vi "总磷总氮通讯.vi"() -> ()   [LabVIEW 2016, in "斯坦道总磷总氮.lvlib"]
uses:
  <vilib>/Plasmionique/MB Master/MB_Master_Serial/MB_Master_Serial.lvclass
  C:/Program Files (x86)/National Instruments/LabVIEW 2016/vi.lib/Plasmionique/MB Master/MB_Master/MB_Master.lvclass
  <vilib>/Plasmionique/MB Master/MB_Master_TCP/MB_Master_TCP.lvclass
  <vilib>/Utility/config.llb/Write Key (Boolean).vi
  <vilib>/Utility/config.llb/Write Key (String).vi
  <vilib>/Plasmionique/MB Master/MB_Master/MB_Master.lvclass
  <vilib>/Utility/config.llb/NI_LVConfig.lvlib
  <vilib>/Plasmionique/MB Master/MB Master.lvlib
  <vilib>/ptbypt/NI_PtbyPt.lvlib
panel:
  out "启用":bool=TRUE
  out "氨氮状态告警区":u16[](array[numeric])
  out "氨氮测量数据区":u16[](array[numeric])
  out "COD测量数据区":u16[](array[numeric])
  out "COD状态告警区":u16[](array[numeric])
  out "总氮测量数据区":u16[](array[numeric])
  out "总氮状态告警区":u16[](array[numeric])
  out "总磷状态告警区":u16[](array[numeric])
  out "总磷测量数据区":u16[](array[numeric])
  out "状态告警区":T1 {"告警代码" items=["无告警", "缺试剂告警", "缺水样告警", "缺蒸馏水告警", "缺标液告警", "仪表漏液告警", "标定异常告警", "超量程告警", "加热异常", "低试剂预警", "超上限告警", "超下限告警", "仪表内部其他异常", "滴定异常告警", "电极异常告警", "量程切换告警", "参数设置告警", "PH电极电位异常", "电导率电极异常", "浊度光度异常", "溶解氧电极异常", "溶解氧光强异常", "温度异常告警", "PH异常告警", "溶解氧异常告警", "电导率异常告警", "浊度异常告警", "叶绿素异常告警", "藻密度异常告警", "蓝绿藻异常告警", "ORP异常告警", "氨氮异常告警", "清洁刷异常告警", "SD卡异常告警", "蓝牙异常告警", "Wifi异常告警", "流程异常告警"]; "故障代码" items=["无故障", "电机故障", "温度故障", "通讯故障", "滴定故障"]}
  out "测量数据区":T2 {"单位" items=["ug/L", "mg/L", "ppm", "mg/m3", "cm", "ppb", "ug/m3", "%", "nmol/mol", "umol/mol", "MPN/L", "MPN/100ml", "ng/m3", "NTU", "无量纲", "ms/cm", "us/cm", "℃", "mV", "万个/L"]}
  out "status":bool
  out "关键参数区":T3
  in  "读关键参数区":bool
  in  "读状态告警区":bool
  in  "读测量数据区":bool
  in  "站号":u16(ring) items=["总磷"=1, "氨氮"=3]
  in  "停止":bool
  in  "启动":bool
  in  "控制命令":u16(ring) items=["启动测量"=1, "标样核查"=2, "零点核查"=3, "跨度核查"=4, "空白测试"=5, "平行样测试"=6, "加标回收"=7, "空白校准"=8, "标样校准"=9, "初始化（清洗）"=10, "停止测试"=11, "仪器重启"=12, "校时"=13, "模式设置"=14, "测量间隔设置"=15]
  in  "控制命令参数":u16[](array[numeric]) format="%04xH"
  in  "VISA Resource":refnum<visa-resource-name>
  in  "启用模块":bool
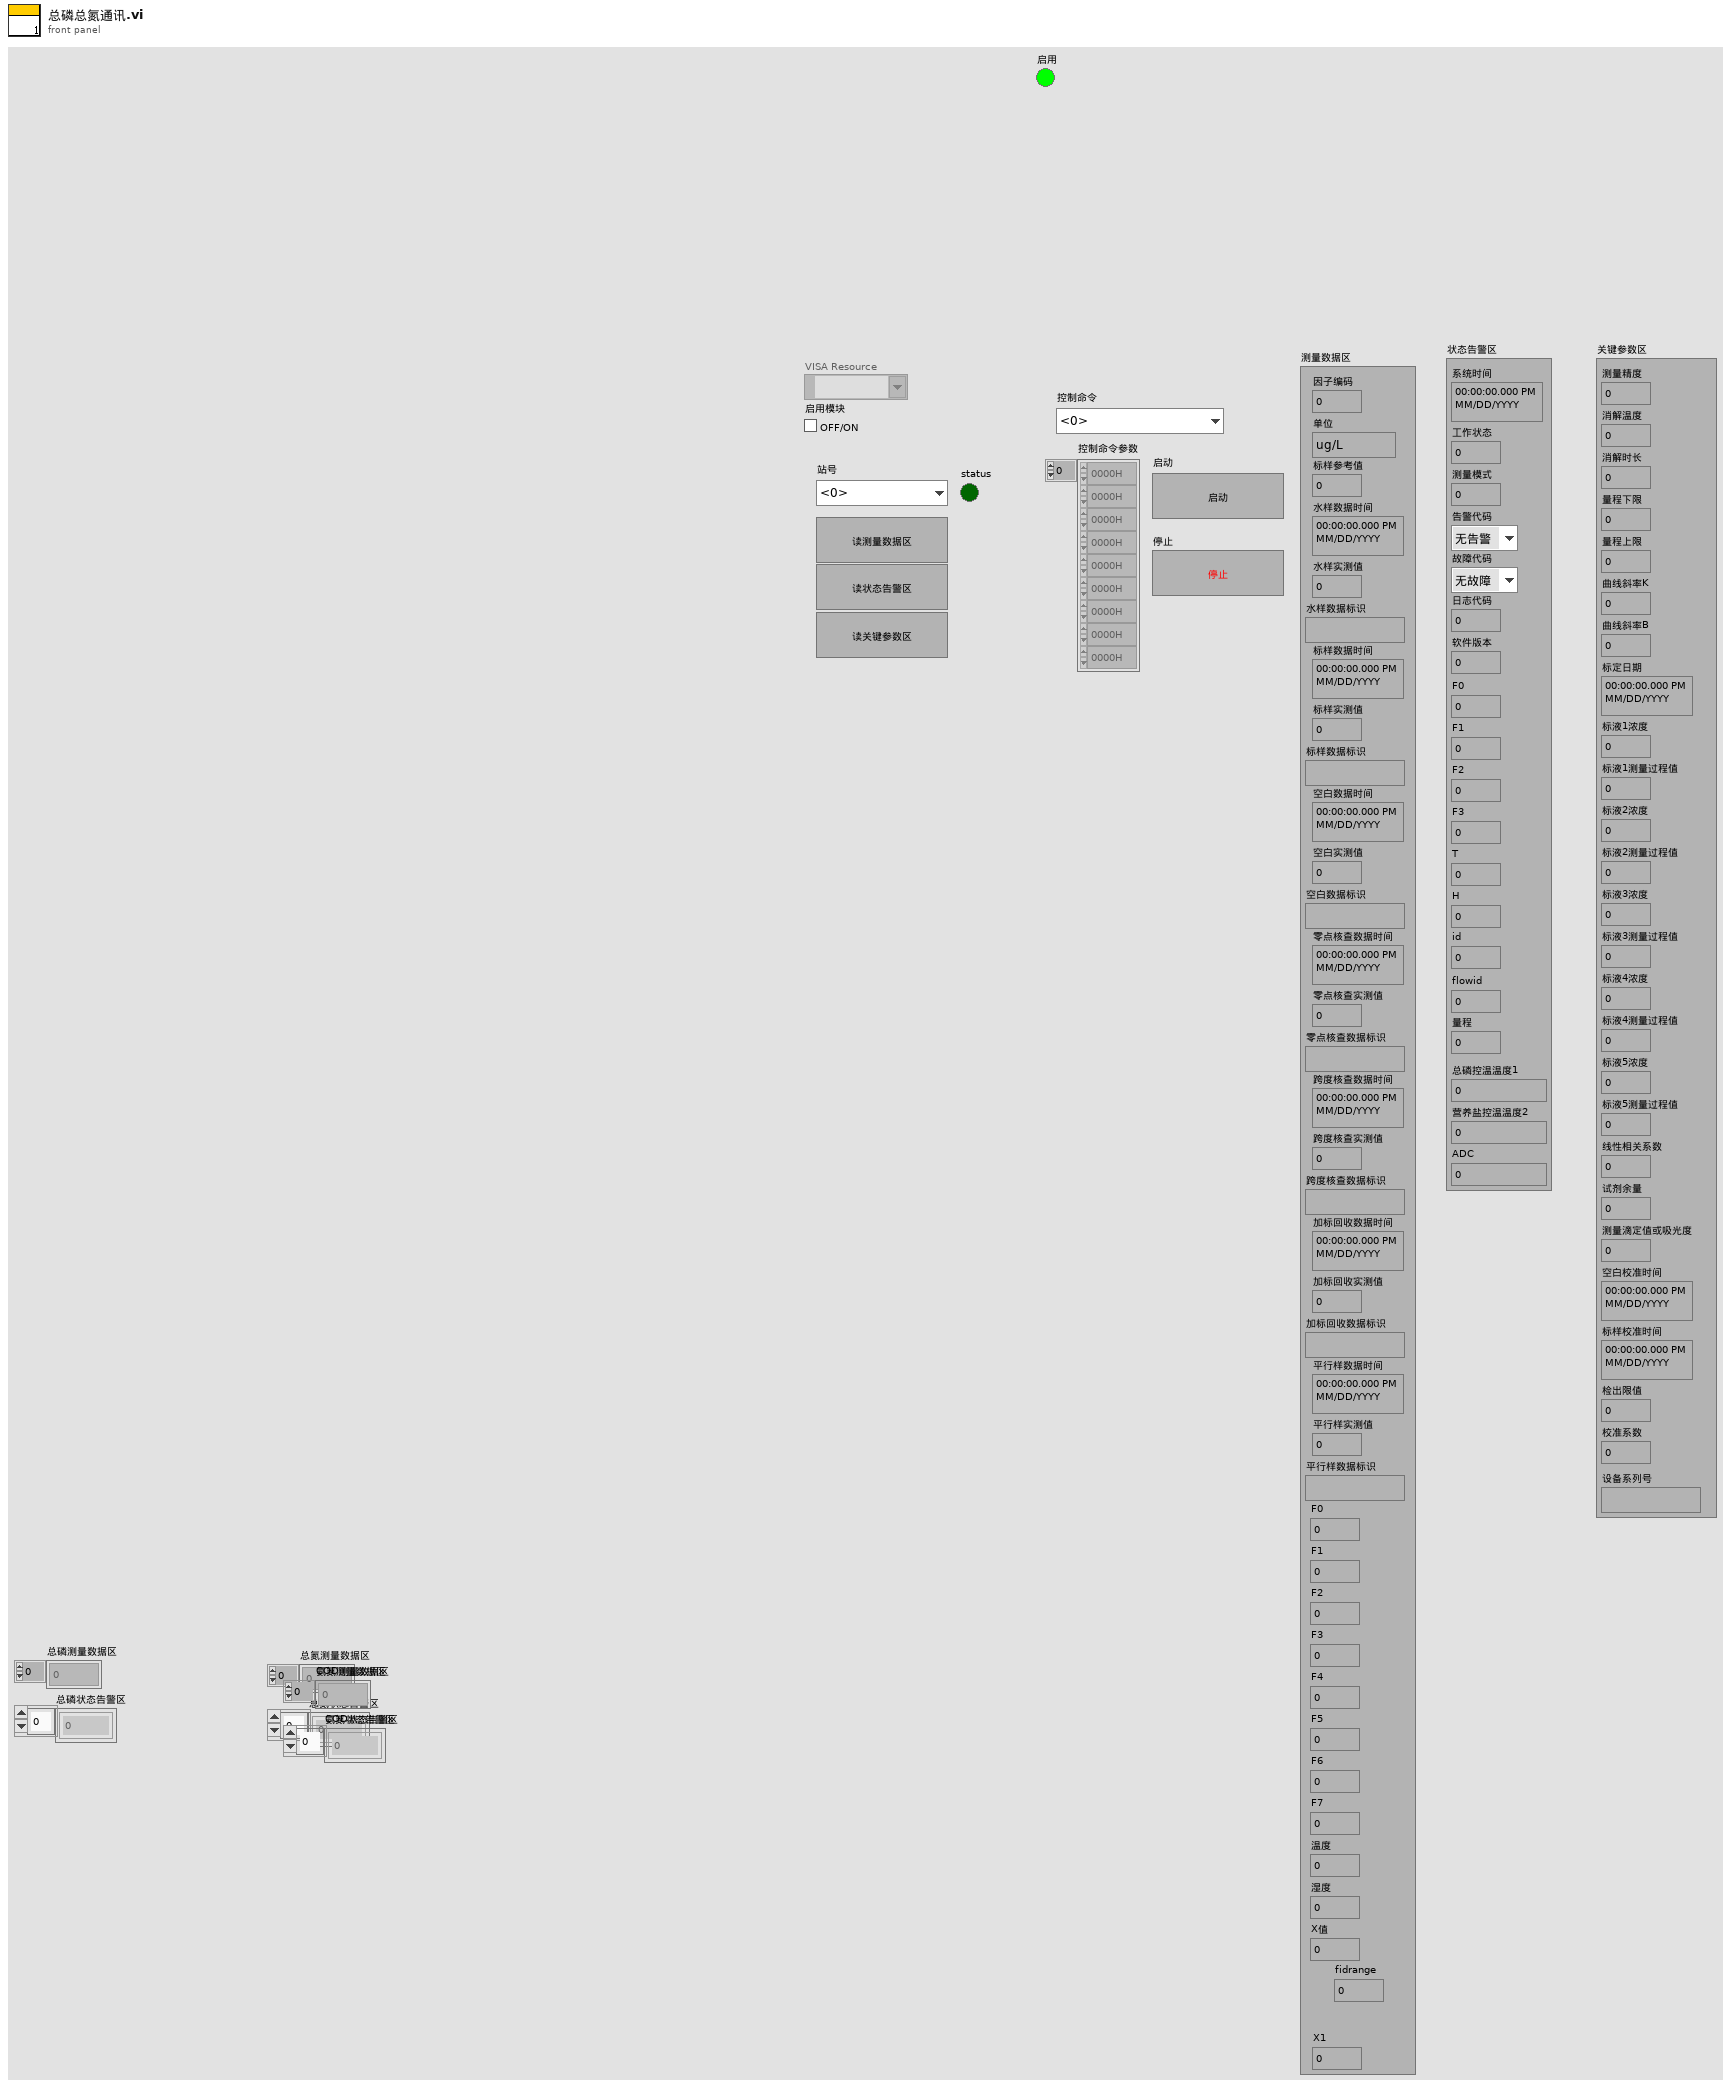
[diagram p1: front panel]
types:
  T1 = cluster{"系统时间":timestamp, "工作状态":u16, "测量模式":u16, "告警代码":u16, "故障代码":u16, "日志代码":u16, "软件版本":u16, "F0":sgl, "F1":sgl, "F2":sgl, "F3":sgl, "T":sgl, "H":sgl, "id":u16, "flowid":u16, "量程":u16, "总磷控温温度1":sgl, "营养盐控温温度2":sgl, "ADC":sgl}
  T2 = cluster{"因子编码":u32, "单位":u16, "标样参考值":sgl, "水样数据时间":timestamp, "水样实测值":sgl, "水样数据标识":string, "标样数据时间":timestamp, "标样实测值":sgl, "标样数据标识":string, "空白数据时间":timestamp, "空白实测值":sgl, "空白数据标识":string, "零点核查数据时间":timestamp, "零点核查实测值":sgl, "零点核查数据标识":string, "跨度核查数据时间":timestamp, "跨度核查实测值":sgl, "跨度核查数据标识":string, "加标回收数据时间":timestamp, "加标回收实测值":sgl, "加标回收数据标识":string, "平行样数据时间":timestamp, "平行样实测值":sgl, "平行样数据标识":string, "F0":sgl, "F1":sgl, "F2":sgl, "F3":sgl, "F4":sgl, "F5":sgl, "F6":sgl, "F7":sgl, "温度":sgl, "湿度":sgl, "X值":sgl, "fidrange":u16, "X1":sgl}
  T3 = cluster{"测量精度":u16, "消解温度":u16, "消解时长":u16, "量程下限":sgl, "量程上限":sgl, "曲线斜率K":sgl, "曲线斜率B":sgl, "标定日期":timestamp, "标液1浓度":sgl, "标液1测量过程值":sgl, "标液2浓度":sgl, "标液2测量过程值":sgl, "标液3浓度":sgl, "标液3测量过程值":sgl, "标液4浓度":sgl, "标液4测量过程值":sgl, "标液5浓度":sgl, "标液5测量过程值":sgl, "线性相关系数":sgl, "试剂余量":u32, "测量滴定值或吸光度":sgl, "空白校准时间":timestamp, "标样校准时间":timestamp, "检出限值":sgl, "校准系数":sgl, "设备系列号":string}
  T4 = cluster{"系统时间":timestamp, "工作状态":u16, "测量模式":enum16{"待机", "连续模式", "周期模式", "定点模式", "受控模式", "手动模式"}, "告警代码":u16, "故障代码":u16, "日志代码":u16, "软件版本":u16, "F0":sgl, "F1":sgl, "F2":sgl, "F3":sgl, "T":sgl, "H":sgl, "id":u16, "flowid":u16, "量程":u16, "总磷控温温度1":sgl, "营养盐控温温度2":sgl, "ADC":sgl}
  T5 = cluster{"因子编码":u32, "单位":u16, "标样参考值":sgl, "水样数据时间":timestamp, "水样实测值":sgl, "水样数据标识":string, "标样数据时间":timestamp, "标样实测值":sgl, "标样数据标识":string, "空白数据时间":timestamp, "空白实测值":sgl, "空白数据标识":string, "零点核查数据时间":timestamp, "零点核查实测值":sgl, "零点核查数据标识":string, "跨度核查数据时间":timestamp, "跨度核查实测值":sgl, "跨度核查数据标识":string, "加标回收数据时间":timestamp, "加标回收实测值":sgl, "加标回收数据标识":string, "平行样数据时间":timestamp, "平行样实测值":sgl, "平行样数据标识":string, "F0":sgl, "F1":sgl, "F2":sgl, "F3":sgl, "F4":sgl, "F5":sgl, "F6":sgl, "F7":sgl, "温度":sgl, "湿度":sgl, "X值":sgl, "fidrange":u16, "X1值":sgl}
  T6 = cluster{"测量精度":u16, "消解温度":u16, "消解时长":u16, "量程下限":sgl, "量程上限":sgl, "曲线斜率K":sgl, "曲线斜率B":sgl, "标定日期":timestamp, "标液1浓度":sgl, "标液1测量过程值":sgl, "标液2浓度":sgl, "标液2测量过程值":sgl, "标液3浓度":sgl, "标液3测量过程值":sgl, "标液4浓度":sgl, "标液4测量过程值":sgl, "标液5浓度":sgl, "标液5测量过程值":sgl, "线性相关系数":sgl, "试剂余量":u32, "测量滴定值或吸光度":sgl, "空白校准时间":timestamp, "标样校准时间":timestamp, "检出限值":sgl, "校准系数":sgl, "设备系列号":string}[]
  T7 = cluster{"系统时间":timestamp, "工作状态":u16, "测量模式":enum16{"待机", "连续模式", "周期模式", "定点模式", "受控模式", "手动模式"}, "告警代码":u16, "故障代码":u16, "日志代码":u16, "软件版本":u16, "F0":sgl, "F1":sgl, "F2":sgl, "F3":sgl, "T":sgl, "H":sgl, "id":u16, "flowid":u16, "量程":u16, "总磷控温温度1":sgl, "营养盐控温温度2":sgl, "ADC":sgl}[]
  T8 = cluster{"因子编码":u32, "单位":u16, "标样参考值":sgl, "水样数据时间":timestamp, "水样实测值":sgl, "水样数据标识":string, "标样数据时间":timestamp, "标样实测值":sgl, "标样数据标识":string, "空白数据时间":timestamp, "空白实测值":sgl, "空白数据标识":string, "零点核查数据时间":timestamp, "零点核查实测值":sgl, "零点核查数据标识":string, "跨度核查数据时间":timestamp, "跨度核查实测值":sgl, "跨度核查数据标识":string, "加标回收数据时间":timestamp, "加标回收实测值":sgl, "加标回收数据标识":string, "平行样数据时间":timestamp, "平行样实测值":sgl, "平行样数据标识":string, "F0":sgl, "F1":sgl, "F2":sgl, "F3":sgl, "F4":sgl, "F5":sgl, "F6":sgl, "F7":sgl, "温度":sgl, "湿度":sgl, "X值":sgl, "fidrange":u16, "X1值":sgl}[]
  T9 = typedef "CODCr交互.ctl" = cluster{"状态告警区":cluster{"系统时间":timestamp, "工作状态":u16, "测量模式":enum16{"待机", "连续模式", "周期模式", "定点模式", "受控模式", "手动模式"}, "告警代码":u16, "故障代码":u16, "日志代码":u16, "软件版本":u16, "F0":sgl, "F1":sgl, "F2":sgl, "F3":sgl, "T":sgl, "H":sgl, "id":u16, "flowid":u16, "量程":u16, "总磷控温温度1":sgl, "营养盐控温温度2":sgl, "ADC":sgl}, "平台试剂余量百分比":sgl, "关键参数":cluster{"测量量程":dbl, "测量精度":dbl, "测量间隔":dbl, "消解温度":dbl, "消解时长":dbl, "空白校准时间":timestamp, "曲线截距":dbl, "曲线斜率":dbl, "测量检出限":dbl, "测量信号值":dbl, "线性相关系数":dbl, "二次多项式系数":dbl, "标样校准时间":timestamp, "稀释倍数":dbl, "三项式系数":dbl, "空白标定系数":dbl, "量程系数":dbl, "F0/ORPA":dbl, "F1/ORPB":dbl, "F2/ORPK":dbl, "F3":dbl, "F4":dbl, "F5":dbl, "F6":dbl, "F7":dbl, "X0/滴定数":dbl, "量程":dbl}, "关键参数改变":bool, "校准信息":cluster{"低标液1浓度":dbl, "低标液1信号值":dbl, "低标液1启用":u16, "低标液2浓度":dbl, "低标液2信号值":dbl, "低标液2启用":u16, "低标液3浓度":dbl, "低标液3信号值":dbl, "低标液3启用":u16, "低标液4浓度":dbl, "低标液4信号值":dbl, "低标液4启用":u16, "低标液5浓度":dbl, "低标液5信号值":dbl, "低标液5启用":u16, "高标液1浓度":dbl, "高标液1信号值":dbl, "高标液1启用":u16, "高标液2浓度":dbl, "高标液2信号值":dbl, "高标液2启用":u16, "高标液3浓度":dbl, "高标液3信号值":dbl, "高标液3启用":u16, "高标液4浓度":dbl, "高标液4信号值":dbl, "高标液4启用":u16, "高标液5浓度":dbl, "高标液5信号值":dbl, "高标液5启用":u16, "低斜率":dbl, "低截距":dbl, "低二次多项式系数":dbl, "低线性相关系数":dbl, "高斜率":dbl, "高截距":dbl, "高二次多项式系数":dbl, "高线性相关系数":dbl}, "校准信息改变":bool}
  T10 = typedef "总磷交互.ctl" = cluster{"状态告警区":cluster{"系统时间":timestamp, "工作状态":u16, "测量模式":enum16{"待机", "连续模式", "周期模式", "定点模式", "受控模式", "手动模式"}, "告警代码":u16, "故障代码":u16, "日志代码":u16, "软件版本":u16, "F0":sgl, "F1":sgl, "F2":sgl, "F3":sgl, "T":sgl, "H":sgl, "id":u16, "flowid":u16, "量程":u16, "总磷控温温度1":sgl, "营养盐控温温度2":sgl, "ADC":sgl}, "平台试剂余量百分比":sgl, "关键参数":cluster{"测量量程":dbl, "测量精度":dbl, "测量间隔":dbl, "消解温度":dbl, "消解时长":dbl, "空白校准时间":timestamp, "曲线截距":dbl, "曲线斜率":dbl, "测量检出限":dbl, "测量信号值":dbl, "线性相关系数":dbl, "二次多项式系数":dbl, "标样校准时间":timestamp, "稀释倍数":dbl, "三项式系数":dbl, "空白标定系数":dbl, "量程系数":dbl, "F0/ORPA":dbl, "F1/ORPB":dbl, "F2/ORPK":dbl, "F3":dbl, "F4":dbl, "F5":dbl, "F6":dbl, "F7":dbl, "X0/滴定数":dbl, "量程":dbl}, "关键参数改变":bool, "校准信息":cluster{"低标液1浓度":dbl, "低标液1信号值":dbl, "低标液1启用":u16, "低标液2浓度":dbl, "低标液2信号值":dbl, "低标液2启用":u16, "低标液3浓度":dbl, "低标液3信号值":dbl, "低标液3启用":u16, "低标液4浓度":dbl, "低标液4信号值":dbl, "低标液4启用":u16, "低标液5浓度":dbl, "低标液5信号值":dbl, "低标液5启用":u16, "高标液1浓度":dbl, "高标液1信号值":dbl, "高标液1启用":u16, "高标液2浓度":dbl, "高标液2信号值":dbl, "高标液2启用":u16, "高标液3浓度":dbl, "高标液3信号值":dbl, "高标液3启用":u16, "高标液4浓度":dbl, "高标液4信号值":dbl, "高标液4启用":u16, "高标液5浓度":dbl, "高标液5信号值":dbl, "高标液5启用":u16, "低斜率":dbl, "低截距":dbl, "低二次多项式系数":dbl, "低线性相关系数":dbl, "高斜率":dbl, "高截距":dbl, "高二次多项式系数":dbl, "高线性相关系数":dbl}, "校准信息改变":bool}
  T11 = typedef "总氮交互.ctl" = cluster{"状态告警区":cluster{"系统时间":timestamp, "工作状态":u16, "测量模式":enum16{"待机", "连续模式", "周期模式", "定点模式", "受控模式", "手动模式"}, "告警代码":u16, "故障代码":u16, "日志代码":u16, "软件版本":u16, "F0":sgl, "F1":sgl, "F2":sgl, "F3":sgl, "T":sgl, "H":sgl, "id":u16, "flowid":u16, "量程":u16, "总磷控温温度1":sgl, "营养盐控温温度2":sgl, "ADC":sgl}, "平台试剂余量百分比":sgl, "关键参数":cluster{"测量量程":dbl, "测量精度":dbl, "测量间隔":dbl, "消解温度":dbl, "消解时长":dbl, "空白校准时间":timestamp, "曲线截距":dbl, "曲线斜率":dbl, "测量检出限":dbl, "测量信号值":dbl, "线性相关系数":dbl, "二次多项式系数":dbl, "标样校准时间":timestamp, "稀释倍数":dbl, "三项式系数":dbl, "空白标定系数":dbl, "量程系数":dbl, "F0/ORPA":dbl, "F1/ORPB":dbl, "F2/ORPK":dbl, "F3":dbl, "F4":dbl, "F5":dbl, "F6":dbl, "F7":dbl, "X0/滴定数":dbl, "量程":dbl}, "关键参数改变":bool, "校准信息":cluster{"低标液1浓度":dbl, "低标液1信号值":dbl, "低标液1启用":u16, "低标液2浓度":dbl, "低标液2信号值":dbl, "低标液2启用":u16, "低标液3浓度":dbl, "低标液3信号值":dbl, "低标液3启用":u16, "低标液4浓度":dbl, "低标液4信号值":dbl, "低标液4启用":u16, "低标液5浓度":dbl, "低标液5信号值":dbl, "低标液5启用":u16, "高标液1浓度":dbl, "高标液1信号值":dbl, "高标液1启用":u16, "高标液2浓度":dbl, "高标液2信号值":dbl, "高标液2启用":u16, "高标液3浓度":dbl, "高标液3信号值":dbl, "高标液3启用":u16, "高标液4浓度":dbl, "高标液4信号值":dbl, "高标液4启用":u16, "高标液5浓度":dbl, "高标液5信号值":dbl, "高标液5启用":u16, "低斜率":dbl, "低截距":dbl, "低二次多项式系数":dbl, "低线性相关系数":dbl, "高斜率":dbl, "高截距":dbl, "高二次多项式系数":dbl, "高线性相关系数":dbl}, "校准信息改变":bool}
  T12 = typedef "氨氮交互.ctl" = cluster{"状态告警区":cluster{"系统时间":timestamp, "工作状态":u16, "测量模式":enum16{"待机", "连续模式", "周期模式", "定点模式", "受控模式", "手动模式"}, "告警代码":u16, "故障代码":u16, "日志代码":u16, "软件版本":u16, "F0":sgl, "F1":sgl, "F2":sgl, "F3":sgl, "T":sgl, "H":sgl, "id":u16, "flowid":u16, "量程":u16, "总磷控温温度1":sgl, "营养盐控温温度2":sgl, "ADC":sgl}, "平台试剂余量百分比":sgl, "关键参数":cluster{"测量量程":dbl, "测量精度":dbl, "测量间隔":dbl, "消解温度":dbl, "消解时长":dbl, "空白校准时间":timestamp, "曲线截距":dbl, "曲线斜率":dbl, "测量检出限":dbl, "测量信号值":dbl, "线性相关系数":dbl, "二次多项式系数":dbl, "标样校准时间":timestamp, "稀释倍数":dbl, "三项式系数":dbl, "空白标定系数":dbl, "量程系数":dbl, "F0/ORPA":dbl, "F1/ORPB":dbl, "F2/ORPK":dbl, "F3":dbl, "F4":dbl, "F5":dbl, "F6":dbl, "F7":dbl, "X0/滴定数":dbl, "量程":dbl}, "关键参数改变":bool, "校准信息":cluster{"低标液1浓度":dbl, "低标液1信号值":dbl, "低标液1启用":u16, "低标液2浓度":dbl, "低标液2信号值":dbl, "低标液2启用":u16, "低标液3浓度":dbl, "低标液3信号值":dbl, "低标液3启用":u16, "低标液4浓度":dbl, "低标液4信号值":dbl, "低标液4启用":u16, "低标液5浓度":dbl, "低标液5信号值":dbl, "低标液5启用":u16, "高标液1浓度":dbl, "高标液1信号值":dbl, "高标液1启用":u16, "高标液2浓度":dbl, "高标液2信号值":dbl, "高标液2启用":u16, "高标液3浓度":dbl, "高标液3信号值":dbl, "高标液3启用":u16, "高标液4浓度":dbl, "高标液4信号值":dbl, "高标液4启用":u16, "高标液5浓度":dbl, "高标液5信号值":dbl, "高标液5启用":u16, "低斜率":dbl, "低截距":dbl, "低二次多项式系数":dbl, "低线性相关系数":dbl, "高斜率":dbl, "高截距":dbl, "高二次多项式系数":dbl, "高线性相关系数":dbl}, "校准信息改变":bool}
  T13 = typedef "NI_LVConfig.lvlib/Config Data RefNum.ctl" = refnum<k1>
  T14 = enum8{"Enabled", "Disabled", "Disabled and Grayed Out"}
  T15 = cluster{"baud rate (bps)":u32, "stop bits":u16, "parity":u16, "flow control":u16, "timeout":u32, "retries":i32}
  T16 = cluster{"测量量程":dbl, "测量精度":dbl, "测量间隔":dbl, "消解温度":dbl, "消解时长":dbl, "空白校准时间":timestamp, "曲线截距":dbl, "曲线斜率":dbl, "测量检出限":dbl, "测量信号值":dbl, "线性相关系数":dbl, "二次多项式系数":dbl, "标样校准时间":timestamp, "稀释倍数":dbl, "三项式系数":dbl, "空白标定系数":dbl, "量程系数":dbl, "F0/ORPA":dbl, "F1/ORPB":dbl, "F2/ORPK":dbl, "F3":dbl, "F4":dbl, "F5":dbl, "F6":dbl, "F7":dbl, "X0/滴定数":dbl, "量程":dbl}
  T17 = typedef "斯坦道总磷总氮.lvlib/关键参数.ctl" = cluster{"测量量程":sgl, "测量检出限":sgl, "测量精度":sgl, "测量间隔":sgl, "消解温度":sgl, "消解时长":sgl, "三项式系数":sgl, "二次多项式系数":sgl, "曲线斜率":sgl, "曲线截距":sgl, "线性相关系数":sgl, "空白校准时间":timestamp, "标样校准时间":timestamp, "测量信号值":sgl, "稀释倍数":sgl, "空白标定系数":sgl, "量程系数":sgl}
  T18 = cluster{"低标液1浓度":dbl, "低标液1信号值":dbl, "低标液1启用":u16, "低标液2浓度":dbl, "低标液2信号值":dbl, "低标液2启用":u16, "低标液3浓度":dbl, "低标液3信号值":dbl, "低标液3启用":u16, "低标液4浓度":dbl, "低标液4信号值":dbl, "低标液4启用":u16, "低标液5浓度":dbl, "低标液5信号值":dbl, "低标液5启用":u16, "高标液1浓度":dbl, "高标液1信号值":dbl, "高标液1启用":u16, "高标液2浓度":dbl, "高标液2信号值":dbl, "高标液2启用":u16, "高标液3浓度":dbl, "高标液3信号值":dbl, "高标液3启用":u16, "高标液4浓度":dbl, "高标液4信号值":dbl, "高标液4启用":u16, "高标液5浓度":dbl, "高标液5信号值":dbl, "高标液5启用":u16, "低斜率":dbl, "低截距":dbl, "低二次多项式系数":dbl, "低线性相关系数":dbl, "高斜率":dbl, "高截距":dbl, "高二次多项式系数":dbl, "高线性相关系数":dbl}
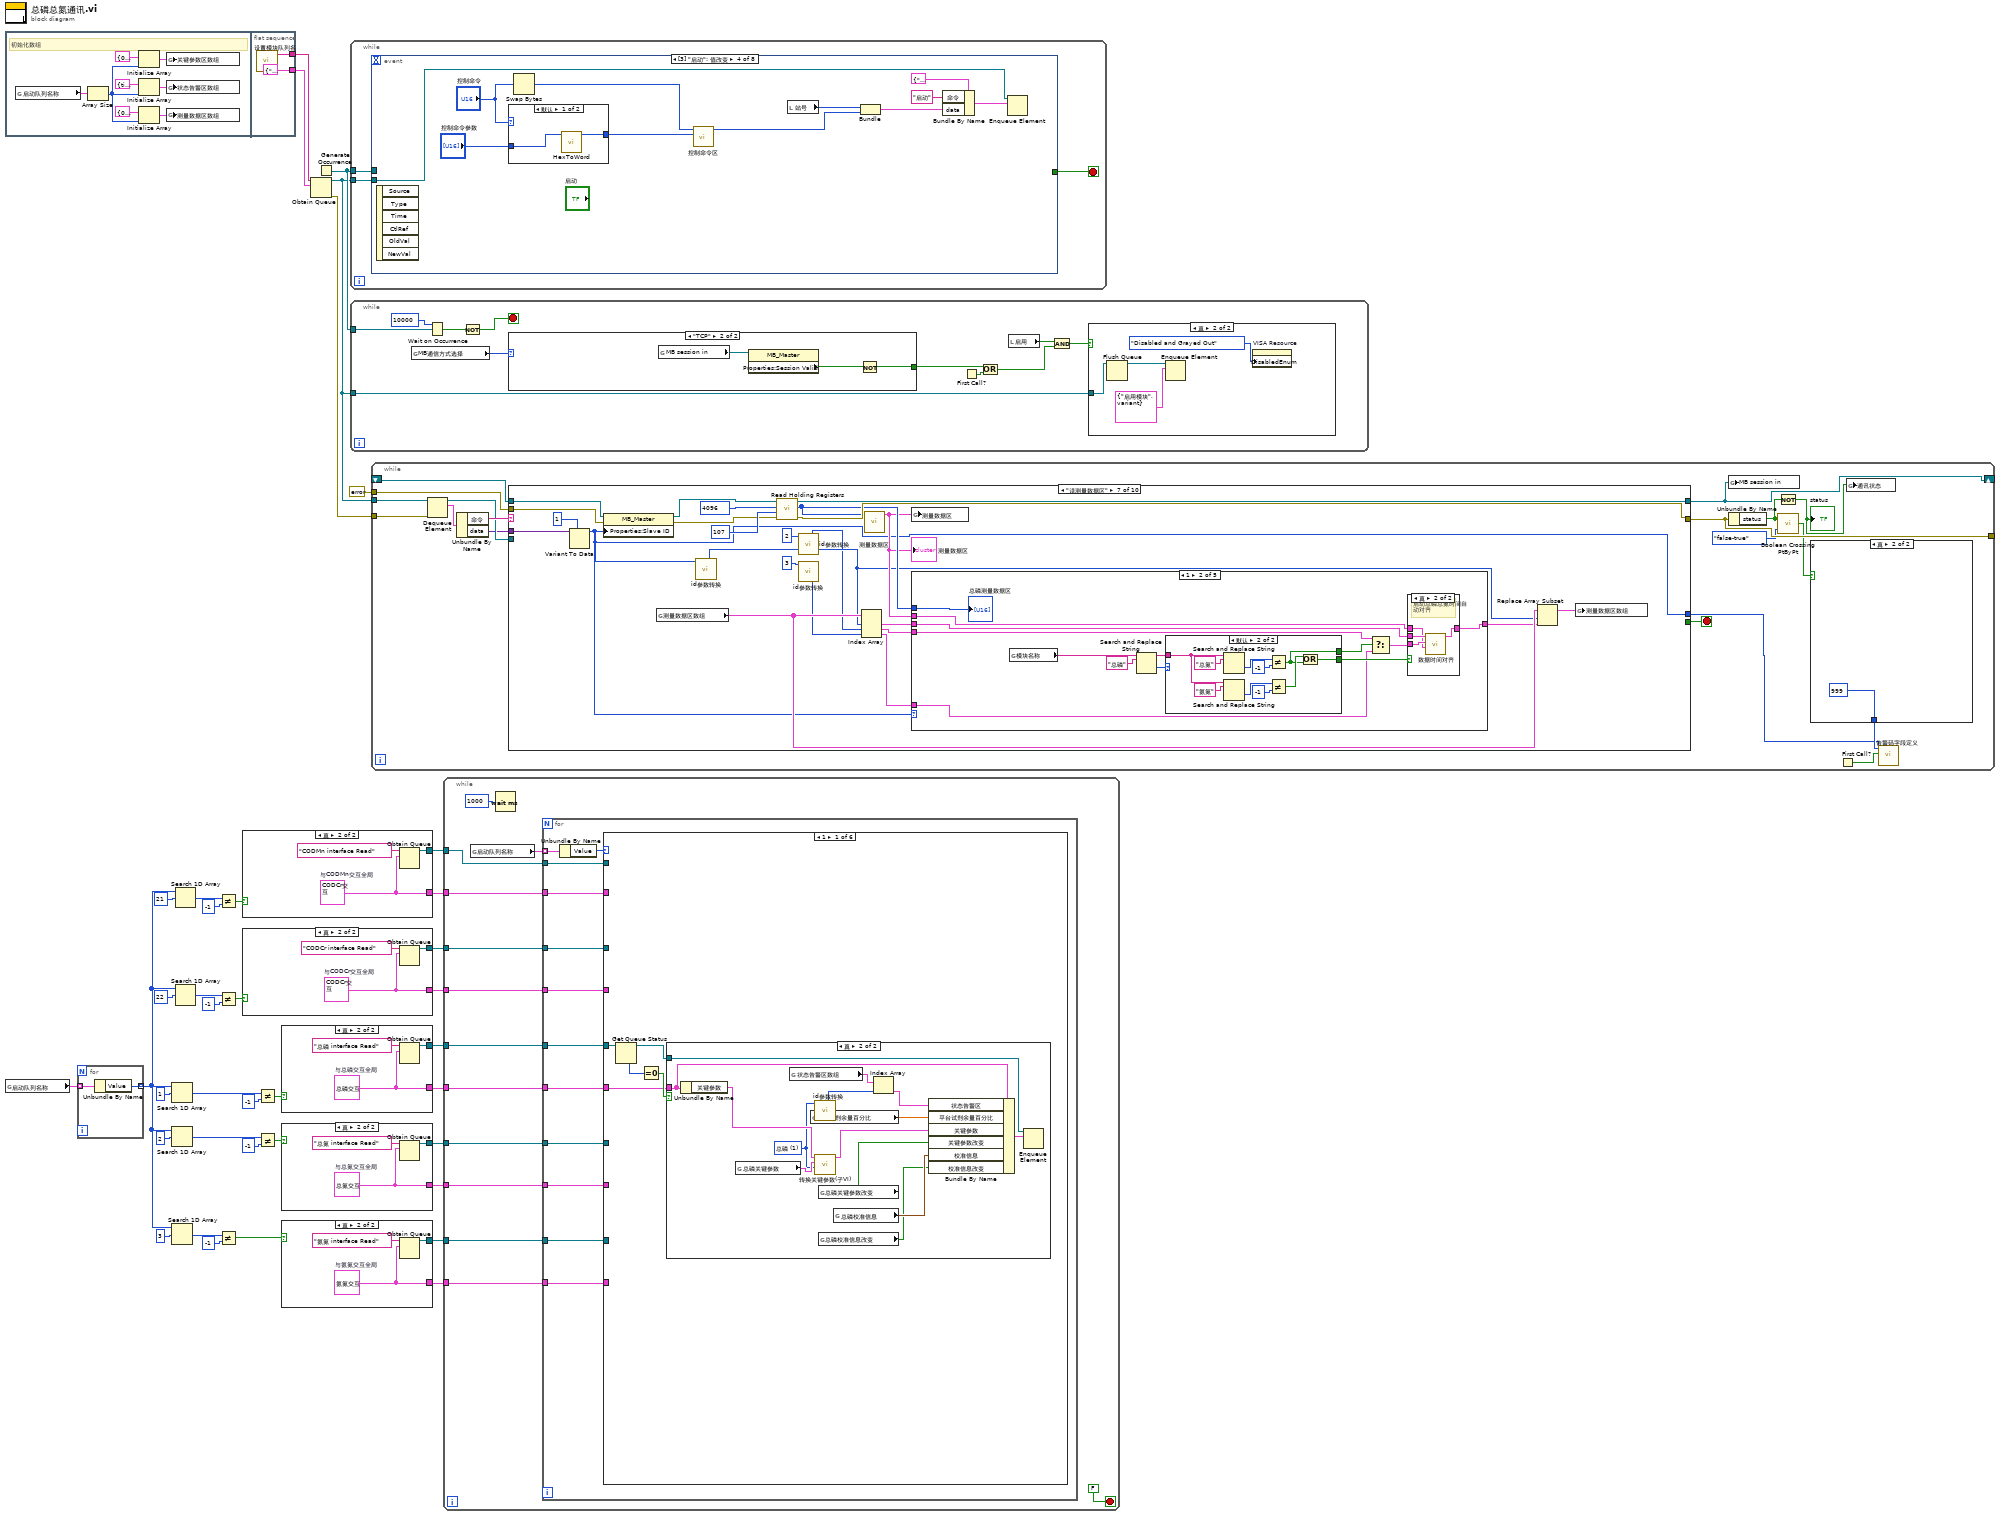
[diagram p0: block diagram]
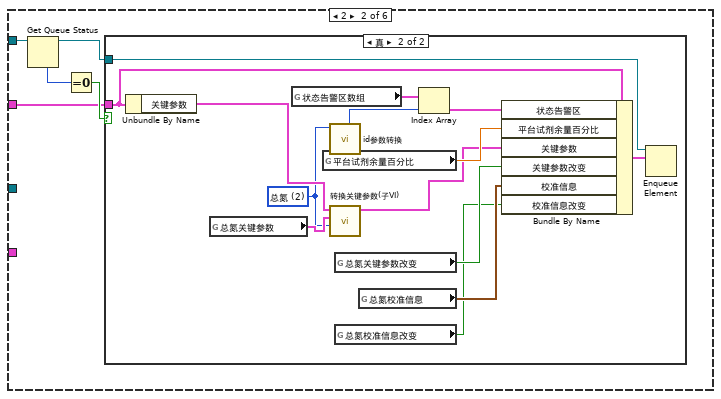
[diagram p8: hidden frame]
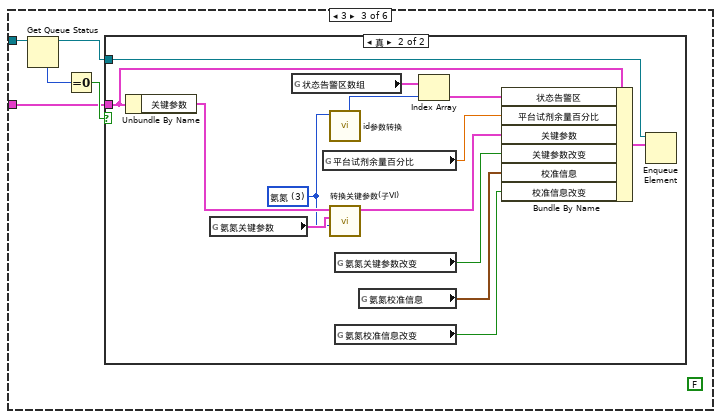
[diagram p10: hidden frame]
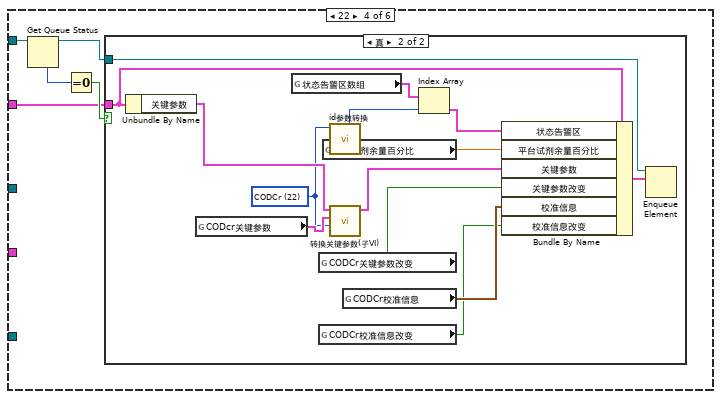
[diagram p12: hidden frame]
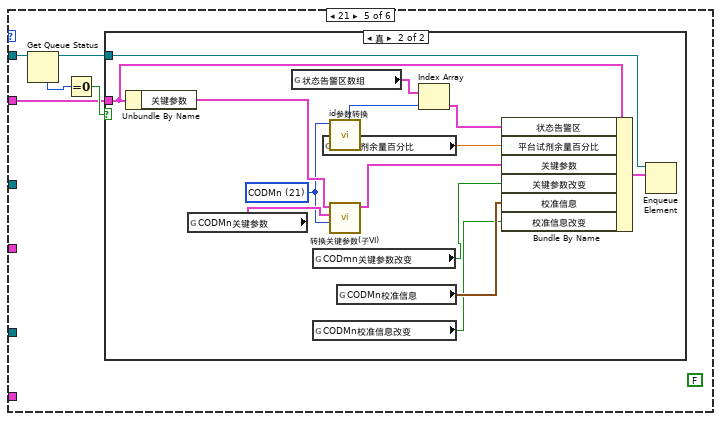
[diagram p14: hidden frame]
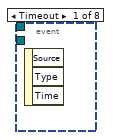
[diagram p19: hidden frame]
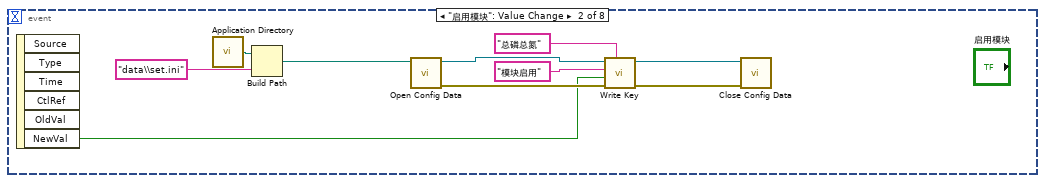
[diagram p20: hidden frame]
diagram:
  n1 = flat-sequence {
    tunnel: [cluster{"命令":string, "data":variant} {"命令"="", "data"=variant}] -> w38
    tunnel: [w47] -> w33
    frame #0 {
      # "初始化数组"
      n2 = global read "model config var.vi" "启动队列名称"() -> (w40:cluster{"String":string, "Value":u16}[])
      n3 = Array Size(array=w40) -> (size(s)=w39:i32)
      n4 = Initialize Array(T3 {"测量精度"=0, "消解温度"=0, "消解时长"=0, "量程下限"=0.0, "量程上限"=0.0, "曲线斜率K"=0.0, "曲线斜率B"=0.0, "标定日期"=timestamp(0 s since 1904-01-01), "标液1浓度"=0.0, "标液1测量过程值"=0.0, "标液2浓度"=0.0, "标液2测量过程值"=0.0, "标液3浓度"=0.0, "标液3测量过程值"=0.0, "标液4浓度"=0.0, "标液4测量过程值"=0.0, "标液5浓度"=0.0, "标液5测量过程值"=0.0, "线性相关系数"=0.0, "试剂余量"=0, "测量滴定值或吸光度"=0.0, "空白校准时间"=timestamp(0 s since 1904-01-01), "标样校准时间"=timestamp(0 s since 1904-01-01), "检出限值"=0.0, "校准系数"=0.0, "设备系列号"=""} ("关键参数区"), w39) -> (w44:T6)
      n5 = Initialize Array(T4 {"系统时间"=timestamp(0 s since 1904-01-01), "工作状态"=0, "测量模式"=enum."待机", "告警代码"=0, "故障代码"=0, "日志代码"=0, "软件版本"=0, "F0"=0.0, "F1"=0.0, "F2"=0.0, "F3"=0.0, "T"=0.0, "H"=0.0, "id"=0, "flowid"=0, "量程"=0, "总磷控温温度1"=0.0, "营养盐控温温度2"=0.0, "ADC"=0.0} ("状态告警区"), w39) -> (w43:T7)
      n6 = Initialize Array(T5 {"因子编码"=0, "单位"=0, "标样参考值"=0.0, "水样数据时间"=timestamp(0 s since 1904-01-01), "水样实测值"=0.0, "水样数据标识"="", "标样数据时间"=timestamp(0 s since 1904-01-01), "标样实测值"=0.0, "标样数据标识"="", "空白数据时间"=timestamp(0 s since 1904-01-01), "空白实测值"=0.0, "空白数据标识"="", "零点核查数据时间"=timestamp(0 s since 1904-01-01), "零点核查实测值"=0.0, "零点核查数据标识"="", "跨度核查数据时间"=timestamp(0 s since 1904-01-01), "跨度核查实测值"=0.0, "跨度核查数据标识"="", "加标回收数据时间"=timestamp(0 s since 1904-01-01), "加标回收实测值"=0.0, "加标回收数据标识"="", "平行样数据时间"=timestamp(0 s since 1904-01-01), "平行样实测值"=0.0, "平行样数据标识"="", "F0"=0.0, "F1"=0.0, "F2"=0.0, "F3"=0.0, "F4"=0.0, "F5"=0.0, "F6"=0.0, "F7"=0.0, "温度"=0.0, "湿度"=0.0, "X值"=0.0, "fidrange"=0, "X1值"=0.0} ("测量数据区"), w39) -> (w46:T8)
      n7 = global write "VAR总磷总氮全局变量.vi" "关键参数区数组"(w44) -> ()
      n8 = global write "VAR总磷总氮全局变量.vi" "状态告警区数组"(w43) -> ()
      n9 = global write "VAR总磷总氮全局变量.vi" "测量数据区数组"(w46) -> ()
    }
    frame #1 {
      n10 = call "设置模块队列名.vi"() -> ("Msg"=w47:string)  [unwired: 5 in]
    }
  }
  n11 = global read "model config var.vi" "启动队列名称"() -> (w22:cluster{"String":string, "Value":u16}[])
  n12 = for {
    tunnel: w22 -> [w50] mode=indexing
    tunnel: [w49] -> w2 mode=indexing
    n13 = Unbundle By Name(w50) -> ("Value"=w49:u16)
  }
  n14 = Search 1D Array(1D array=w2, element=u16 1 ("元素")) -> (index of element=w12:i32)  [unwired: 1 in]
  n15 = Search 1D Array(1D array=w2, element=u16 2 ("元素")) -> (index of element=w8:i32)  [unwired: 1 in]
  n16 = Search 1D Array(1D array=w2, element=u16 3 ("元素")) -> (index of element=w4:i32)  [unwired: 1 in]
  n17 = Search 1D Array(1D array=w2, element=u16 21 ("元素")) -> (index of element=w20:i32)  [unwired: 1 in]
  n18 = Search 1D Array(1D array=w2, element=u16 22 ("元素")) -> (index of element=w16:i32)  [unwired: 1 in]
  n19 = Not Equal?(x=w20, y=-1) -> (x != y?=w18:bool)
  n20 = Not Equal?(x=w16, y=-1) -> (x != y?=w14:bool)
  n21 = Not Equal?(x=w4, y=-1) -> (x != y?=w1:bool)
  n22 = case shown="真" w18 {
    tunnel: [_ w52] -> w32
    tunnel: [_ w51] -> w31
    frame False {
    }
    frame True {
      w51 = T9 {"状态告警区"={"系统时间"=timestamp(0 s since 1904-01-01), "工作状态"=0, "测量模式"=enum."待机", "告警代码"=0, "故障代码"=0, "日志代码"=0, "软件版本"=0, "F0"=0.0, "F1"=0.0, "F2"=0.0, "F3"=0.0, "T"=0.0, "H"=0.0, "id"=0, "flowid"=0, "量程"=0, "总磷控温温度1"=0.0, "营养盐控温温度2"=0.0, "ADC"=0.0}, "平台试剂余量百分比"=0.0, "关键参数"={"测量量程"=0.0, "测量精度"=0.0, "测量间隔"=0.0, "消解温度"=0.0, "消解时长"=0.0, "空白校准时间"=timestamp(0 s since 1904-01-01), "曲线截距"=0.0, "曲线斜率"=0.0, "测量检出限"=0.0, "测量信号值"=0.0, "线性相关系数"=0.0, "二次多项式系数"=0.0, "标样校准时间"=timestamp(0 s since 1904-01-01), "稀释倍数"=0.0, "三项式系数"=0.0, "空白标定系数"=0.0, "量程系数"=0.0, "F0/ORPA"=0.0, "F1/ORPB"=0.0, "F2/ORPK"=0.0, "F3"=0.0, "F4"=0.0, "F5"=0.0, "F6"=0.0, "F7"=0.0, "X0/滴定数"=0.0, "量程"=0.0}, "关键参数改变"=FALSE, "校准信息"={"低标液1浓度"=0.0, "低标液1信号值"=0.0, "低标液1启用"=0, "低标液2浓度"=0.0, "低标液2信号值"=0.0, "低标液2启用"=0, "低标液3浓度"=0.0, "低标液3信号值"=0.0, "低标液3启用"=0, "低标液4浓度"=0.0, "低标液4信号值"=0.0, "低标液4启用"=0, "低标液5浓度"=0.0, "低标液5信号值"=0.0, "低标液5启用"=0, "高标液1浓度"=0.0, "高标液1信号值"=0.0, "高标液1启用"=0, "高标液2浓度"=0.0, "高标液2信号值"=0.0, "高标液2启用"=0, "高标液3浓度"=0.0, "高标液3信号值"=0.0, "高标液3启用"=0, "高标液4浓度"=0.0, "高标液4信号值"=0.0, "高标液4启用"=0, "高标液5浓度"=0.0, "高标液5信号值"=0.0, "高标液5启用"=0, "低斜率"=0.0, "低截距"=0.0, "低二次多项式系数"=0.0, "低线性相关系数"=0.0, "高斜率"=0.0, "高截距"=0.0, "高二次多项式系数"=0.0, "高线性相关系数"=0.0}, "校准信息改变"=FALSE}  # 与CODMn交互全局
      n23 = Obtain Queue(name (unnamed)="CODMn interface Read" ("写入方名称"), element data type=w51) -> (queue out=w52:refnum<queue>)  [unwired: 3 in, 2 out]
    }
  }
  n24 = case shown="真" w14 {
    tunnel: [_ w55] -> w30
    tunnel: [_ w54] -> w29
    frame False {
    }
    frame True {
      w54 = T9 {"状态告警区"={"系统时间"=timestamp(0 s since 1904-01-01), "工作状态"=0, "测量模式"=enum."待机", "告警代码"=0, "故障代码"=0, "日志代码"=0, "软件版本"=0, "F0"=0.0, "F1"=0.0, "F2"=0.0, "F3"=0.0, "T"=0.0, "H"=0.0, "id"=0, "flowid"=0, "量程"=0, "总磷控温温度1"=0.0, "营养盐控温温度2"=0.0, "ADC"=0.0}, "平台试剂余量百分比"=0.0, "关键参数"={"测量量程"=0.0, "测量精度"=0.0, "测量间隔"=0.0, "消解温度"=0.0, "消解时长"=0.0, "空白校准时间"=timestamp(0 s since 1904-01-01), "曲线截距"=0.0, "曲线斜率"=0.0, "测量检出限"=0.0, "测量信号值"=0.0, "线性相关系数"=0.0, "二次多项式系数"=0.0, "标样校准时间"=timestamp(0 s since 1904-01-01), "稀释倍数"=0.0, "三项式系数"=0.0, "空白标定系数"=0.0, "量程系数"=0.0, "F0/ORPA"=0.0, "F1/ORPB"=0.0, "F2/ORPK"=0.0, "F3"=0.0, "F4"=0.0, "F5"=0.0, "F6"=0.0, "F7"=0.0, "X0/滴定数"=0.0, "量程"=0.0}, "关键参数改变"=FALSE, "校准信息"={"低标液1浓度"=0.0, "低标液1信号值"=0.0, "低标液1启用"=0, "低标液2浓度"=0.0, "低标液2信号值"=0.0, "低标液2启用"=0, "低标液3浓度"=0.0, "低标液3信号值"=0.0, "低标液3启用"=0, "低标液4浓度"=0.0, "低标液4信号值"=0.0, "低标液4启用"=0, "低标液5浓度"=0.0, "低标液5信号值"=0.0, "低标液5启用"=0, "高标液1浓度"=0.0, "高标液1信号值"=0.0, "高标液1启用"=0, "高标液2浓度"=0.0, "高标液2信号值"=0.0, "高标液2启用"=0, "高标液3浓度"=0.0, "高标液3信号值"=0.0, "高标液3启用"=0, "高标液4浓度"=0.0, "高标液4信号值"=0.0, "高标液4启用"=0, "高标液5浓度"=0.0, "高标液5信号值"=0.0, "高标液5启用"=0, "低斜率"=0.0, "低截距"=0.0, "低二次多项式系数"=0.0, "低线性相关系数"=0.0, "高斜率"=0.0, "高截距"=0.0, "高二次多项式系数"=0.0, "高线性相关系数"=0.0}, "校准信息改变"=FALSE}  # 与CODCr交互全局
      n25 = Obtain Queue(name (unnamed)="CODCr interface Read" ("写入方名称"), element data type=w54) -> (queue out=w55:refnum<queue>)  [unwired: 3 in, 2 out]
    }
  }
  n26 = Not Equal?(x=w12, y=-1) -> (x != y?=w10:bool)
  n27 = Not Equal?(x=w8, y=-1) -> (x != y?=w6:bool)
  n28 = case shown="真" w10 {
    tunnel: [_ w58] -> w28
    tunnel: [_ w57] -> w27
    frame False {
    }
    frame True {
      w57 = T10 {"状态告警区"={"系统时间"=timestamp(0 s since 1904-01-01), "工作状态"=0, "测量模式"=enum."待机", "告警代码"=0, "故障代码"=0, "日志代码"=0, "软件版本"=0, "F0"=0.0, "F1"=0.0, "F2"=0.0, "F3"=0.0, "T"=0.0, "H"=0.0, "id"=0, "flowid"=0, "量程"=0, "总磷控温温度1"=0.0, "营养盐控温温度2"=0.0, "ADC"=0.0}, "平台试剂余量百分比"=0.0, "关键参数"={"测量量程"=0.0, "测量精度"=0.0, "测量间隔"=0.0, "消解温度"=0.0, "消解时长"=0.0, "空白校准时间"=timestamp(0 s since 1904-01-01), "曲线截距"=0.0, "曲线斜率"=0.0, "测量检出限"=0.0, "测量信号值"=0.0, "线性相关系数"=0.0, "二次多项式系数"=0.0, "标样校准时间"=timestamp(0 s since 1904-01-01), "稀释倍数"=0.0, "三项式系数"=0.0, "空白标定系数"=0.0, "量程系数"=0.0, "F0/ORPA"=0.0, "F1/ORPB"=0.0, "F2/ORPK"=0.0, "F3"=0.0, "F4"=0.0, "F5"=0.0, "F6"=0.0, "F7"=0.0, "X0/滴定数"=0.0, "量程"=0.0}, "关键参数改变"=FALSE, "校准信息"={"低标液1浓度"=0.0, "低标液1信号值"=0.0, "低标液1启用"=0, "低标液2浓度"=0.0, "低标液2信号值"=0.0, "低标液2启用"=0, "低标液3浓度"=0.0, "低标液3信号值"=0.0, "低标液3启用"=0, "低标液4浓度"=0.0, "低标液4信号值"=0.0, "低标液4启用"=0, "低标液5浓度"=0.0, "低标液5信号值"=0.0, "低标液5启用"=0, "高标液1浓度"=0.0, "高标液1信号值"=0.0, "高标液1启用"=0, "高标液2浓度"=0.0, "高标液2信号值"=0.0, "高标液2启用"=0, "高标液3浓度"=0.0, "高标液3信号值"=0.0, "高标液3启用"=0, "高标液4浓度"=0.0, "高标液4信号值"=0.0, "高标液4启用"=0, "高标液5浓度"=0.0, "高标液5信号值"=0.0, "高标液5启用"=0, "低斜率"=0.0, "低截距"=0.0, "低二次多项式系数"=0.0, "低线性相关系数"=0.0, "高斜率"=0.0, "高截距"=0.0, "高二次多项式系数"=0.0, "高线性相关系数"=0.0}, "校准信息改变"=FALSE}  # 与总磷交互全局
      n29 = Obtain Queue(name (unnamed)="总磷 interface Read" ("写入方名称"), element data type=w57) -> (queue out=w58:refnum<queue>)  [unwired: 3 in, 2 out]
    }
  }
  n30 = case shown="真" w6 {
    tunnel: [_ w61] -> w26
    tunnel: [_ w60] -> w25
    frame False {
    }
    frame True {
      w60 = T11 {"状态告警区"={"系统时间"=timestamp(0 s since 1904-01-01), "工作状态"=0, "测量模式"=enum."待机", "告警代码"=0, "故障代码"=0, "日志代码"=0, "软件版本"=0, "F0"=0.0, "F1"=0.0, "F2"=0.0, "F3"=0.0, "T"=0.0, "H"=0.0, "id"=0, "flowid"=0, "量程"=0, "总磷控温温度1"=0.0, "营养盐控温温度2"=0.0, "ADC"=0.0}, "平台试剂余量百分比"=0.0, "关键参数"={"测量量程"=0.0, "测量精度"=0.0, "测量间隔"=0.0, "消解温度"=0.0, "消解时长"=0.0, "空白校准时间"=timestamp(0 s since 1904-01-01), "曲线截距"=0.0, "曲线斜率"=0.0, "测量检出限"=0.0, "测量信号值"=0.0, "线性相关系数"=0.0, "二次多项式系数"=0.0, "标样校准时间"=timestamp(0 s since 1904-01-01), "稀释倍数"=0.0, "三项式系数"=0.0, "空白标定系数"=0.0, "量程系数"=0.0, "F0/ORPA"=0.0, "F1/ORPB"=0.0, "F2/ORPK"=0.0, "F3"=0.0, "F4"=0.0, "F5"=0.0, "F6"=0.0, "F7"=0.0, "X0/滴定数"=0.0, "量程"=0.0}, "关键参数改变"=FALSE, "校准信息"={"低标液1浓度"=0.0, "低标液1信号值"=0.0, "低标液1启用"=0, "低标液2浓度"=0.0, "低标液2信号值"=0.0, "低标液2启用"=0, "低标液3浓度"=0.0, "低标液3信号值"=0.0, "低标液3启用"=0, "低标液4浓度"=0.0, "低标液4信号值"=0.0, "低标液4启用"=0, "低标液5浓度"=0.0, "低标液5信号值"=0.0, "低标液5启用"=0, "高标液1浓度"=0.0, "高标液1信号值"=0.0, "高标液1启用"=0, "高标液2浓度"=0.0, "高标液2信号值"=0.0, "高标液2启用"=0, "高标液3浓度"=0.0, "高标液3信号值"=0.0, "高标液3启用"=0, "高标液4浓度"=0.0, "高标液4信号值"=0.0, "高标液4启用"=0, "高标液5浓度"=0.0, "高标液5信号值"=0.0, "高标液5启用"=0, "低斜率"=0.0, "低截距"=0.0, "低二次多项式系数"=0.0, "低线性相关系数"=0.0, "高斜率"=0.0, "高截距"=0.0, "高二次多项式系数"=0.0, "高线性相关系数"=0.0}, "校准信息改变"=FALSE}  # 与总氮交互全局
      n31 = Obtain Queue(name (unnamed)="总氮 interface Read" ("写入方名称"), element data type=w60) -> (queue out=w61:refnum<queue>)  [unwired: 3 in, 2 out]
    }
  }
  n32 = case shown="真" w1 {
    tunnel: [_ w64] -> w24
    tunnel: [_ w63] -> w23
    frame False {
    }
    frame True {
      w63 = T12 {"状态告警区"={"系统时间"=timestamp(0 s since 1904-01-01), "工作状态"=0, "测量模式"=enum."待机", "告警代码"=0, "故障代码"=0, "日志代码"=0, "软件版本"=0, "F0"=0.0, "F1"=0.0, "F2"=0.0, "F3"=0.0, "T"=0.0, "H"=0.0, "id"=0, "flowid"=0, "量程"=0, "总磷控温温度1"=0.0, "营养盐控温温度2"=0.0, "ADC"=0.0}, "平台试剂余量百分比"=0.0, "关键参数"={"测量量程"=0.0, "测量精度"=0.0, "测量间隔"=0.0, "消解温度"=0.0, "消解时长"=0.0, "空白校准时间"=timestamp(0 s since 1904-01-01), "曲线截距"=0.0, "曲线斜率"=0.0, "测量检出限"=0.0, "测量信号值"=0.0, "线性相关系数"=0.0, "二次多项式系数"=0.0, "标样校准时间"=timestamp(0 s since 1904-01-01), "稀释倍数"=0.0, "三项式系数"=0.0, "空白标定系数"=0.0, "量程系数"=0.0, "F0/ORPA"=0.0, "F1/ORPB"=0.0, "F2/ORPK"=0.0, "F3"=0.0, "F4"=0.0, "F5"=0.0, "F6"=0.0, "F7"=0.0, "X0/滴定数"=0.0, "量程"=0.0}, "关键参数改变"=FALSE, "校准信息"={"低标液1浓度"=0.0, "低标液1信号值"=0.0, "低标液1启用"=0, "低标液2浓度"=0.0, "低标液2信号值"=0.0, "低标液2启用"=0, "低标液3浓度"=0.0, "低标液3信号值"=0.0, "低标液3启用"=0, "低标液4浓度"=0.0, "低标液4信号值"=0.0, "低标液4启用"=0, "低标液5浓度"=0.0, "低标液5信号值"=0.0, "低标液5启用"=0, "高标液1浓度"=0.0, "高标液1信号值"=0.0, "高标液1启用"=0, "高标液2浓度"=0.0, "高标液2信号值"=0.0, "高标液2启用"=0, "高标液3浓度"=0.0, "高标液3信号值"=0.0, "高标液3启用"=0, "高标液4浓度"=0.0, "高标液4信号值"=0.0, "高标液4启用"=0, "高标液5浓度"=0.0, "高标液5信号值"=0.0, "高标液5启用"=0, "低斜率"=0.0, "低截距"=0.0, "低二次多项式系数"=0.0, "低线性相关系数"=0.0, "高斜率"=0.0, "高截距"=0.0, "高二次多项式系数"=0.0, "高线性相关系数"=0.0}, "校准信息改变"=FALSE}  # 与氨氮交互全局
      n33 = Obtain Queue(name (unnamed)="氨氮 interface Read" ("写入方名称"), element data type=w63) -> (queue out=w64:refnum<queue>)  [unwired: 3 in, 2 out]
    }
  }
  n34 = Obtain Queue(name (unnamed)=w33, element data type=w38) -> (queue out=w34:refnum<queue>, error out=w37:errorcluster)  [unwired: 3 in, 1 out]
  n35 = Generate Occurrence() -> (w35:refnum<k4>)
  n36 = while {
    tunnel: w34 -> [w68]
    tunnel: w35 -> [w66]
    stop <- w67 stop-if-true
    n37 = event shown="[3] \"启动\": 值改变" {
      selector: _ -> [_ _ _ _ _ _ _ _]
      dyn-events: _ -> [_ _ _ _ _ _ _ _]
      timeout: _ -> [_ _ _ _ _ _ _ _]
      tunnel: w68 -> [_ _ _ w99 w106 w112 w117 w122]
      tunnel: [_ _ _ _ "停止" _ _ _] -> w67
      tunnel: w66 -> [_ _ _ _ w103 _ _ _]
      event Timeout {
        n38 = event-data() -> ()  [unwired: 1 in, 3 out]
      }
      event "启用模块": Value Change {
        n39 = event-data() -> ("NewVal"=w69:bool)  [unwired: 1 in, 5 out]
        n40 = call <vilib>:"Application Directory.vi"() -> ("Application Directory"=w71:path)
        n41 = Build Path(base path=w71, name or relative path="data\\set.ini" ("名称或相对路径")) -> (appended path=w72:path)
        n42 = call <vilib>:"Open Config Data.vi"("configuration file path"=w72) -> ("error out"=w78:errorcluster, "refnum"=w77:T13)  [unwired: 8 in, 1 out]
        n43 = call-poly <vilib>:"Write Key.vi"("section"="总磷总氮", "error in (no error)"=w78, "value"=w69, "key"="模块启用", "refnum"=w77) -> ("error out"=w74:errorcluster, "refnum out"=w70:T13)  [unwired: 4 in, 1 out]
        n44 = call <vilib>:"Close Config Data.vi"("error in (no error)"=w74, "refnum"=w70) -> ()  [unwired: 8 in, 2 out]
      }
      event "VISA Resource": Value Change {
        n45 = event-data() -> ()  [unwired: 1 in, 6 out]
        n46 = call <vilib>:"Application Directory.vi"() -> ("Application Directory"=w81:path)
        n47 = Build Path(base path=w81, name or relative path="data\\set.ini" ("名称或相对路径")) -> (appended path=w82:path)
        n48 = call <vilib>:"Open Config Data.vi"("configuration file path"=w82) -> ("error out"=w88:errorcluster, "refnum"=w87:T13)  [unwired: 8 in, 1 out]
        n49 = call-poly <vilib>:"Write Key.vi"("section"="总磷总氮", "error in (no error)"=w88, "value"="VISA Resource", "key"="串口", "refnum"=w87) -> ("error out"=w84:errorcluster, "refnum out"=w80:T13)  [unwired: 4 in, 1 out]
        n50 = call <vilib>:"Close Config Data.vi"("error in (no error)"=w84, "refnum"=w80) -> ()  [unwired: 8 in, 2 out]
      }
      event "启动": Value Change {
        n51 = event-data() -> ()  [unwired: 1 in, 6 out]
        n52 = case shown="默认" "控制命令" {
          tunnel: "控制命令参数" -> [w101 w102]
          tunnel: [w100 w102] -> w89
          frame Default {
            n53 = call "HexToWord.vi"("数组"=w101) -> ("WORD"=w100:u16[])  [unwired: 10 in]
          }
          frame 13 {
          }
        }
        n54 = Swap Bytes(anything="控制命令") -> (byte swapped=w92:u16)
        n55 = call "控制命令区.vi"("控制命令参数"=w89, "控制命令"=w92) -> ("控制命令"=w95:u16[])  [unwired: 9 in]
        n56 = local read "站号"() -> (w94:u16)
        n57 = Bundle("站号"=w94, "控制命令"=w95) -> (w93:cluster{"站号":u16, "控制命令":u16[]})  [unwired: 1 in]
        n58 = Bundle By Name(cluster=cluster{"命令":string, "data":variant} {"命令"="", "data"=variant} ("元素"), "命令"="启动", "data"=w93) -> (w97:cluster{"命令":string, "data":variant})
        n59 = Enqueue Element(queue=w99, element=w97) -> ()  [unwired: 2 in, 3 out]
      }
      event "停止": Value Change {
        n60 = event-data() -> ()  [unwired: 1 in, 6 out]
        n61 = Set Occurrence(w103) -> ()
        n62 = Flush Queue(queue=w106) -> (queue out=w105:refnum<queue>)  [unwired: 1 in, 2 out]
        n63 = Enqueue Element(queue=w105, element=cluster{"命令":string, "data":variant} {"命令"="shutdown", "data"=variant} ("元素")) -> ()  [unwired: 2 in, 3 out]
      }
      event "读测量数据区": Value Change {
        n64 = event-data() -> ()  [unwired: 1 in, 6 out]
        n65 = Bundle By Name(cluster=cluster{"命令":string, "data":variant} {"命令"="", "data"=variant} ("元素"), "命令"="读测量数据区", "data"="站号") -> (w110:cluster{"命令":string, "data":variant})
        n66 = Enqueue Element(queue=w112, element=w110) -> ()  [unwired: 2 in, 3 out]
      }
      event "读状态告警区": Value Change {
        n67 = event-data() -> ()  [unwired: 1 in, 6 out]
        n68 = local read "站号"() -> (w113:u16)
        n69 = Bundle By Name(cluster=cluster{"命令":string, "data":variant} {"命令"="", "data"=variant} ("元素"), "命令"="读状态告警区", "data"=w113) -> (w115:cluster{"命令":string, "data":variant})
        n70 = Enqueue Element(queue=w117, element=w115) -> ()  [unwired: 2 in, 3 out]
      }
      event "读关键参数区": Value Change {
        n71 = event-data() -> ()  [unwired: 1 in, 6 out]
        n72 = local read "站号"() -> (w118:u16)
        n73 = Bundle By Name(cluster=cluster{"命令":string, "data":variant} {"命令"="", "data"=variant} ("元素"), "命令"="读关键参数区", "data"=w118) -> (w120:cluster{"命令":string, "data":variant})
        n74 = Enqueue Element(queue=w122, element=w120) -> ()  [unwired: 2 in, 3 out]
      }
    }
  }
  n75 = while {
    tunnel: w35 -> [w133]
    tunnel: w34 -> [w129]
    stop <- w130 stop-if-true
    n76 = global read "总磷总氮断电保存全局变量.vi" "MB通信方式选择"() -> (w128:enum16{"串口", "TCP"})
    n77 = Wait on Occurrence(2:w133, 3:10000 ("毫秒超时(-1)")) -> (0:w131:bool)  [unwired: 1 in]
    n78 = Not(x=w131) -> (.not. x?=w130:bool)
    n79 = case shown="\"TCP\"" w128 {
      tunnel: [_ w134] -> w125
      frame "串口", Default {
      }
      frame "TCP" {
        n80 = global read "VAR总磷总氮全局变量.vi" "MB session in"() -> (w136:refnum<class "MB_Master.lvclass">)
        n81 = property class="MB_Master"(reference=w136) -> ("Properties:Session Valid"=w135:bool)  [unwired: 1 in, 2 out]
        n82 = Not(x=w135) -> (.not. x?=w134:bool)
      }
    }
    n83 = First Call?() -> (First Call?: T/F=w127:bool)
    n84 = Or(x=w125, y=w127) -> (x .or. y?=w126:bool)
    n85 = local read "启用"() -> (w123:bool)
    n86 = And(x=w123, y=w126) -> (x .and. y?=w124:bool)
    n87 = case shown="真" w124 {
      tunnel: w129 -> [_ w139]
      frame False {
      }
      frame True {
        n88 = Flush Queue(queue=w139) -> (queue out=w137:refnum<queue>)  [unwired: 1 in, 2 out]
        n89 = Enqueue Element(queue=w137, element=cluster{"命令":string, "data":variant} {"命令"="启用模块", "data"=variant} ("元素")) -> ()  [unwired: 2 in, 3 out]
        n90 = property on="VISA Resource" class="VISAName"("DisabledEnum"=T14."Disabled and Grayed Out" ("禁用")) -> ()  [unwired: 2 in, 2 out]
      }
    }
  }
  n91 = while {
    tunnel: w34 -> [w158]
    tunnel: w37 -> [w157]
    shift-right: [w144] -> _
    shift-left: _ -> [w155]
    tunnel: errorcluster {"status"=FALSE, "code"=0, "source"=""} ("error out") -> [w154]
    tunnel: [w150] -> _
    stop <- w156 stop-if-true
    n92 = Dequeue Element(queue=w158, error in (no error)=w157) -> (queue out=w151:refnum<queue>, element=w152:cluster{"命令":string, "data":variant})  [unwired: 1 in, 2 out]
    n93 = Unbundle By Name(w152) -> ("命令"=w153:string, "data"=w148:variant)
    n94 = case shown="\"读测量数据区\"" w153 {
      tunnel: w148 -> [_ _ _ w193 w204 w221 w242 w291 w311 _]
      tunnel: w151 -> [_ _ _ _ _ _ _ _ _ w324]
      tunnel: [_ _ _ _ _ _ _ _ _ TRUE] -> w156
      tunnel: [w161 w164 w180 w196 w207 w223 w246 w299 w318 w320] -> w144
      tunnel: [w162 w163 w181 w195 w206 w222 w247 w290 w319 w321] -> w150
      tunnel: w155 -> [w161 _ w180 w192 w203 w220 w241 w294 w314 w320]
      tunnel: w154 -> [w162 _ w182 w189 w200 w217 w239 w295 w315 w322]
      tunnel: [_ _ _ w184 w197 w211 w230 w284 w305 _] -> w141
      frame Default {
      }
      frame "启用模块" {
        n95 = global read "总磷总氮断电保存全局变量.vi" "MB通信方式选择"() -> (w165:enum16{"串口", "TCP"})
        n96 = case shown="\"TCP\"" w165 {
          tunnel: [w170 w176] -> w163
          tunnel: [w167 w175] -> w164
          frame "串口", Default {
            n97 = global read "总磷总氮断电保存全局变量.vi" "VISA Resource"() -> (w168:refnum<visa-resource-name>)
            n98 = call <vilib>:"Open Serial Session.vi"("Mode (RTU)"=enum16{"RTU", "ASCII"}."RTU", "Slave ID"=u8 1, "Serial Config"=T15 {"baud rate (bps)"=115200, "stop bits"=10, "parity"=0, "flow control"=0, "timeout"=1000, "retries"=1}, "VISA Resource"=w168) -> ("Error out"=w170:errorcluster, "MB_Serial session"=w167:refnum<class "MB_Master_Serial.lvclass">)  [unwired: 6 in]
          }
          frame "TCP" {
            n99 = global read "总磷总氮断电保存全局变量.vi" "PORT"() -> (w174:string)
            n100 = Decimal String To Number(string=w174) -> (number=w177:i32)  [unwired: 2 in, 1 out]
            n101 = global read "总磷总氮断电保存全局变量.vi" "IP"() -> (w173:string)
            n102 = call <vilib>:"Open TCP Session.vi"("Port (502)"=w177, "IP Address"=w173) -> ("error out"=w176:errorcluster, "MB_TCP session"=w175:refnum<class "MB_Master_TCP.lvclass">)  [unwired: 8 in]
          }
        }
        "启用" <- TRUE
      }
      frame "停用模块" {
        n103 = call-dynamic "Close Session.vi"("error in (no error)"=w182, "MB session in"=w180) -> ("error out"=w178:errorcluster)  [unwired: 9 in]
        n104 = local write "启用"(FALSE ("启用")) -> ()
        n105 = call <vilib>:"Clear Errors.vi"("error in (no error)"=w178) -> ("error out"=w181:errorcluster)  [unwired: 5 in, 1 out]
      }
      frame "启动" {
        n106 = Variant To Data(type=cluster{"站号":u16, "控制命令":u16[]} {"站号"=0, "控制命令"=[]} ("输出簇"), Variant=w193) -> (data=w187:cluster{"站号":u16, "控制命令":u16[]})  [unwired: 1 in, 1 out]
        n107 = Unbundle By Name(w187) -> ("站号"=w184:u16, "控制命令"=w185:u16[])
        n108 = property class="MB_Master"(reference=w192, error in=w189, "Properties:Slave ID"=w184) -> (reference out=w191:refnum<class "MB_Master.lvclass">, error out=w190:errorcluster)
        n109 = Index Array(array=w185) -> (element=w186:u16)  [unwired: 1 in]
        n110 = Swap Bytes(anything=w186) -> (byte swapped=w183:u16)
        n111 = global write "VAR总磷总氮全局变量.vi" "控制命令"(w183) -> ()
        n112 = call <vilib>:"Write Multiple Registers.vi"("error in (no error)"=w190, "values"=w185, "starting address"=u16 4608, "MB session in"=w191) -> ("error out"=w195:errorcluster, "MB session out"=w196:refnum<class "MB_Master.lvclass">)  [unwired: 6 in]
      }
      frame "盲样测试" {
        n113 = Variant To Data(type=u8 0, Variant=w204) -> (data=w197:u8)  [unwired: 1 in, 1 out]
        n114 = property class="MB_Master"(reference=w203, error in=w200, "Properties:Slave ID"=w197) -> (reference out=w202:refnum<class "MB_Master.lvclass">, error out=w201:errorcluster)
        n115 = case shown="默认" w197 {
          tunnel: [u16[] [] ("values") u16[] [33539, 0] ("values") u16[] [23555, 0] ("values")] -> w199
          frame Default {
          }
          frame 1 {
            # "总磷盲样测试命令"
          }
          frame 3 {
            # "氨氮盲样测试"
          }
        }
        n116 = call <vilib>:"Write Multiple Registers.vi"("error in (no error)"=w201, "values"=w199, "starting address"=u16 24592, "MB session in"=w202) -> ("error out"=w206:errorcluster, "MB session out"=w207:refnum<class "MB_Master.lvclass">)  [unwired: 6 in]
      }
      frame "debug" {
        n117 = Variant To Data(type=cluster{"站号":u16, "控制命令":u16[]} {"站号"=0, "控制命令"=[]} ("输出簇"), Variant=w221) -> (data=w215:cluster{"站号":u16, "控制命令":u16[]})  [unwired: 1 in, 1 out]
        n118 = Unbundle By Name(w215) -> ("站号"=w211:u16, "控制命令"=w213:u16[])
        n119 = property class="MB_Master"(reference=w220, error in=w217, "Properties:Slave ID"=w211) -> (reference out=w219:refnum<class "MB_Master.lvclass">, error out=w218:errorcluster)
        n120 = Index Array(array=w213) -> (element=w214:u16)  [unwired: 1 in]
        n121 = global write "VAR总磷总氮全局变量.vi" "控制命令"(w214) -> ()
        n122 = call <vilib>:"Write Multiple Registers.vi"("error in (no error)"=w218, "values"=w213, "starting address"=u16 24594, "MB session in"=w219) -> ("error out"=w222:errorcluster, "MB session out"=w223:refnum<class "MB_Master.lvclass">)  [unwired: 6 in]
      }
      frame "读测量数据区" {
        n123 = Variant To Data(type=u8 1 ("Slave ID"), Variant=w242) -> (data=w230:u8)  [unwired: 1 in, 1 out]
        n124 = property class="MB_Master"(reference=w241, error in=w239, "Properties:Slave ID"=w230) -> (reference out=w240:refnum<class "MB_Master.lvclass">, error out=w238:errorcluster)
        n125 = global read "VAR总磷总氮全局变量.vi" "测量数据区数组"() -> (w235:T8)
        n126 = call "id参数转换.vi"("id"=w230) -> ("数组资源索引"=w229:i32)  [unwired: 9 in, 1 out]
        n127 = call <vilib>:"Read Holding Registers.vi"("error in (no error)"=w238, "quantity"=u16 107, "starting address"=u16 4096, "MB session in"=w240) -> ("error out"=w247:errorcluster, "Registers"=w237:u16[], "MB session out"=w246:refnum<class "MB_Master.lvclass">)  [unwired: 5 in]
        n128 = call "id参数转换.vi"("id"=u16 2) -> ("数组资源索引"=w226:i32)  [unwired: 9 in, 1 out]
        n129 = call "id参数转换.vi"("id"=u16 3) -> ("数组资源索引"=w224:i32)  [unwired: 9 in, 1 out]
        n130 = Index Array(array=w235, index #1=w229, index #2=w226, index #3=w224) -> (element #1=w236:T5, element #2=w231:T5, element #3=w228:T5)
        n131 = call "测量数据区.vi"("数组"=w237) -> ("测量数据区"=w234:T5)  [unwired: 10 in]
        "测量数据区" <- w234
        n132 = global write "VAR总磷总氮全局变量.vi" "测量数据区"(w234) -> ()
        n133 = case shown="1" w230 {
          tunnel: w234 -> [w248 w253 w277 w279 w281]
          tunnel: w237 -> [_ w261 w278 w280 w282]
          tunnel: w236 -> [_ w254 _ _ _]
          tunnel: [w248 w256 w277 w279 w281] -> w233
          tunnel: w231 -> [_ w251 _ _ _]
          tunnel: w228 -> [_ w250 _ _ _]
          frame 0, Default {
          }
          frame 1 {
            n134 = global read "VAR总磷总氮全局变量.vi" "模块名称"() -> (w260:string)
            n135 = Search and Replace String(input string=w260, search string="总磷" ("搜索字符串")) -> (result string=w257:string, offset past replacement=w258:i32)  [unwired: 6 in, 2 out]
            n136 = case shown="默认" w258 {
              tunnel: w257 -> [_ w267]
              tunnel: [_ w264] -> w255
              tunnel: [_ w262] -> w252
              frame -1 {
              }
              frame Default {
                n137 = Search and Replace String(input string=w267, search string="总氮" ("搜索字符串")) -> (offset past replacement=w270:i32)  [unwired: 6 in, 3 out]
                n138 = Search and Replace String(input string=w267, search string="氨氮" ("搜索字符串")) -> (offset past replacement=w265:i32)  [unwired: 6 in, 3 out]
                n139 = Not Equal?(x=w270, y=-1) -> (x != y?=w262:bool)
                n140 = Not Equal?(x=w265, y=-1) -> (x != y?=w263:bool)
                n141 = Or(x=w263, y=w262) -> (x .or. y?=w264:bool)
              }
            }
            n142 = Select(t=w251, s=w252, f=w250) -> (s? t:f=w249:T5)
            n143 = case shown="真" w255 {
              tunnel: [w272 w276] -> w256
              tunnel: w254 -> [_ w275]
              tunnel: w249 -> [_ w274]
              tunnel: w253 -> [w272 w273]
              frame False {
              }
              frame True {
                # "启动总磷总氮时间自动对齐"
                n144 = call "数据时间对齐.vi"("待对齐时间"=w273, "对齐参考时间"=w274, "已对齐时间输入"=w275) -> ("已对齐时间输出"=w276:T5)  [unwired: 8 in]
              }
            }
            "总磷测量数据区" <- w261
          }
          frame 2 {
            "总氮测量数据区" <- w278
          }
          frame 3 {
            "氨氮测量数据区" <- w280
          }
          frame 22 {
            "COD测量数据区" <- w282
          }
        }
        n145 = Replace Array Subset(array=w235, new element=w233, index=w229) -> (w232:T8)
        n146 = global write "VAR总磷总氮全局变量.vi" "测量数据区数组"(w232) -> ()
      }
      frame "读状态告警区" {
        n147 = Variant To Data(type=u8 1 ("Slave ID"), Variant=w291) -> (data=w284:u8)  [unwired: 1 in, 1 out]
        n148 = property class="MB_Master"(reference=w294, error in=w295, "Properties:Slave ID"=w284) -> (reference out=w293:refnum<class "MB_Master.lvclass">, error out=w292:errorcluster)
        n149 = call "id参数转换.vi"("id"=w284) -> ("数组资源索引"=w283:i32)  [unwired: 9 in, 1 out]
        n150 = call <vilib>:"Read Holding Registers.vi"("error in (no error)"=w292, "quantity"=u16 29, "starting address"=u16 4224, "MB session in"=w293) -> ("error out"=w290:errorcluster, "Registers"=w288:u16[], "MB session out"=w299:refnum<class "MB_Master.lvclass">)  [unwired: 5 in]
        n151 = global read "VAR总磷总氮全局变量.vi" "状态告警区数组"() -> (w287:T7)
        n152 = call "状态告警区.vi"("数组"=w288) -> ("状态告警区"=w286:T4)  [unwired: 10 in]
        "状态告警区" <- w286
        n153 = global write "VAR总磷总氮全局变量.vi" "状态告警区"(w286) -> ()
        n154 = Unbundle By Name(w286) -> ("id"=w289:u16)
        n155 = Replace Array Subset(array=w287, new element=w286, index=w283) -> (w285:T7)
        n156 = global write "VAR总磷总氮全局变量.vi" "状态告警区数组"(w285) -> ()
        n157 = case shown="3" w289 {
          tunnel: w286 -> [_ _ _ _ _]
          tunnel: w288 -> [_ w300 w301 w302 w303]
          frame 0, Default {
          }
          frame 1, 131 {
            "总磷状态告警区" <- w300
          }
          frame 2, 76 {
            "总氮状态告警区" <- w301
          }
          frame 3 {
            "氨氮状态告警区" <- w302
          }
          frame 22 {
            "COD状态告警区" <- w303
          }
        }
      }
      frame "读关键参数区" {
        n158 = Variant To Data(type=u8 1 ("Slave ID"), Variant=w311) -> (data=w305:u8)  [unwired: 1 in, 1 out]
        n159 = property class="MB_Master"(reference=w314, error in=w315, "Properties:Slave ID"=w305) -> (reference out=w313:refnum<class "MB_Master.lvclass">, error out=w312:errorcluster)
        n160 = call "id参数转换.vi"("id"=w305) -> ("数组资源索引"=w304:i32)  [unwired: 9 in, 1 out]
        n161 = call <vilib>:"Read Holding Registers.vi"("error in (no error)"=w312, "quantity"=u16 19, "starting address"=u16 4256, "MB session in"=w313) -> ("error out"=w319:errorcluster, "Registers"=w309:u16[], "MB session out"=w318:refnum<class "MB_Master.lvclass">)  [unwired: 5 in]
        n162 = global read "VAR总磷总氮全局变量.vi" "关键参数区数组"() -> (w308:T6)
        n163 = call "关键参数区.vi"("数组"=w309) -> ("关键参数区"=w307:T3)  [unwired: 10 in]
        "关键参数区" <- w307
        n164 = global write "VAR总磷总氮全局变量.vi" "关键参数区"(w307) -> ()
        n165 = Replace Array Subset(array=w308, new element=w307, index=w304) -> (w306:T6)
        n166 = global write "VAR总磷总氮全局变量.vi" "关键参数区数组"(w306) -> ()
      }
      frame "shutdown" {
        n167 = call-dynamic "Close Session.vi"("error in (no error)"=w322, "MB session in"=w320) -> ("error out"=w321:errorcluster)  [unwired: 9 in]
        n168 = Flush Queue(queue=w324) -> (queue out=w323:refnum<queue>)  [unwired: 1 in, 2 out]
        n169 = Release Queue(queue=w323) -> ()  [unwired: 2 in, 3 out]
      }
    }
    n170 = global write "VAR总磷总氮全局变量.vi" "MB session in"(w144) -> ()
    n171 = Unbundle By Name(w150) -> ("status"=w147:bool)
    n172 = Not(x=w147) -> (.not. x?=w149:bool)
    "status" <- w149
    n173 = call <vilib>:"Boolean Crossing PtByPt.vi"("direction"=enum16{"either", "false-true", "true-false"}."false-true", "input"=w147) -> ("crossing"=w146:bool)  [unwired: 1 in]
    n174 = case shown="真" w146 {
      tunnel: [u16 0 ("告警代码") u16 999 ("告警代码")] -> w142
      frame False {
      }
      frame True {
      }
    }
    n175 = First Call?() -> (First Call?: T/F=w143:bool)
    n176 = global write "VAR总磷总氮全局变量.vi" "通讯状态"(w149) -> ()
    n177 = call "告警码字段定义.vi"("id"=w141, "首次调用？"=w143, "告警代码"=w142) -> ()  [unwired: 8 in, 1 out]
  }
  n178 = while {
    tunnel: w32 -> [w335]
    tunnel: w31 -> [w334]
    tunnel: w30 -> [w333]
    tunnel: w29 -> [w332]
    tunnel: w28 -> [w331]
    tunnel: w27 -> [w330]
    tunnel: w26 -> [w329]
    tunnel: w25 -> [w328]
    tunnel: w24 -> [w327]
    tunnel: w23 -> [w326]
    stop <- FALSE stop-if-true
    n179 = global read "model config var.vi" "启动队列名称"() -> (w338:cluster{"String":string, "Value":u16}[])
    n180 = Wait (ms)(milliseconds to wait=u32 1000 ("等待时间（毫秒）")) -> ()  [unwired: 1 out]
    n181 = for {
      tunnel: w338 -> [w350] mode=indexing
      tunnel: w335 -> [w348]
      tunnel: w334 -> [w347]
      tunnel: w333 -> [w346]
      tunnel: w332 -> [w345]
      tunnel: w331 -> [w344]
      tunnel: w330 -> [w343]
      tunnel: w329 -> [w342]
      tunnel: w328 -> [w341]
      tunnel: w327 -> [w340]
      tunnel: w326 -> [w339]
      n182 = Unbundle By Name(w350) -> ("Value"=w349:u16)
      n183 = case shown="1" w349 {
        tunnel: w348 -> [_ _ _ _ w428 _]
        tunnel: w347 -> [_ _ _ _ w427 _]
        tunnel: w346 -> [_ _ _ w409 _ _]
        tunnel: w345 -> [_ _ _ w408 _ _]
        tunnel: w344 -> [w352 _ _ _ _ _]
        tunnel: w343 -> [w351 _ _ _ _ _]
        tunnel: w342 -> [_ w371 _ _ _ _]
        tunnel: w341 -> [_ w370 _ _ _ _]
        tunnel: w340 -> [_ _ w390 _ _ _]
        tunnel: w339 -> [_ _ w389 _ _ _]
        frame 1 {
          n184 = Get Queue Status(queue=w352) -> (queue out=w355:refnum<queue>, # elements in queue=w354:i32)  [unwired: 2 in, 6 out]
          n185 = Equal To 0?(x=w354) -> (x = 0?=w353:bool)
          n186 = case shown="真" w353 {
            tunnel: w351 -> [_ w366]
            tunnel: w355 -> [_ w367]
            frame False {
            }
            frame True {
              w357 = u16 1 items=["总磷"=1, "总氮"=2, "氨氮"=3, "磷酸盐"=4, "硝氮"=5, "亚硝氮"=6, "硅酸盐"=7, "硫化物"=8, "CODCr"=22]
              n187 = Unbundle By Name(w366) -> ("关键参数"=w364:T16)
              n188 = global read "VAR总磷总氮全局变量.vi" "总磷关键参数"() -> (w365:T17)
              n189 = global read "VAR总磷总氮全局变量.vi" "状态告警区数组"() -> (w359:T7)
              n190 = global read "VAR总磷总氮全局变量.vi" "平台试剂余量百分比"() -> (w369:sgl)
              n191 = call "id参数转换.vi"("id"=w357) -> ("数组资源索引"=w358:i32)  [unwired: 9 in, 1 out]
              n192 = call "转换关键参数(子VI).vi"("参数"=w357, "总磷关键参数"=w365, "关键参数输入"=w364) -> ("关键参数输出"=w363:T16)  [unwired: 8 in]
              n193 = global read "VAR总磷总氮全局变量.vi" "总磷关键参数改变"() -> (w362:bool)
              n194 = global read "VAR总磷总氮全局变量.vi" "总磷校准信息改变"() -> (w360:bool)
              n195 = global read "VAR总磷总氮全局变量.vi" "总磷校准信息"() -> (w361:T18)
              n196 = Index Array(array=w359, index=w358) -> (element=w356:T4)
              n197 = Bundle By Name(cluster=w366, "状态告警区"=w356, "平台试剂余量百分比"=w369, "关键参数"=w363, "关键参数改变"=w362, "校准信息"=w361, "校准信息改变"=w360) -> (w368:T10)
              n198 = Enqueue Element(queue=w367, element=w368) -> ()  [unwired: 2 in, 3 out]
            }
          }
        }
        frame 2 {
          n199 = Get Queue Status(queue=w371) -> (queue out=w374:refnum<queue>, # elements in queue=w373:i32)  [unwired: 2 in, 6 out]
          n200 = Equal To 0?(x=w373) -> (x = 0?=w372:bool)
          n201 = case shown="真" w372 {
            tunnel: w374 -> [_ w386]
            tunnel: w370 -> [_ w384]
            frame False {
            }
            frame True {
              w376 = u16 2 items=["总磷"=1, "总氮"=2, "氨氮"=3, "磷酸盐"=4, "硝氮"=5, "亚硝氮"=6, "硅酸盐"=7, "硫化物"=8, "CODCr"=22]
              n202 = Unbundle By Name(w384) -> ("关键参数"=w383:T16)
              n203 = global read "VAR总磷总氮全局变量.vi" "总氮关键参数"() -> (w385:T17)
              n204 = global read "VAR总磷总氮全局变量.vi" "状态告警区数组"() -> (w377:T7)
              n205 = global read "VAR总磷总氮全局变量.vi" "平台试剂余量百分比"() -> (w388:sgl)
              n206 = call "id参数转换.vi"("id"=w376) -> ("数组资源索引"=w378:i32)  [unwired: 9 in, 1 out]
              n207 = call "转换关键参数(子VI).vi"("参数"=w376, "总磷关键参数"=w385, "关键参数输入"=w383) -> ("关键参数输出"=w382:T16)  [unwired: 8 in]
              n208 = global read "VAR总磷总氮全局变量.vi" "总氮关键参数改变"() -> (w381:bool)
              n209 = global read "VAR总磷总氮全局变量.vi" "总氮校准信息改变"() -> (w379:bool)
              n210 = global read "VAR总磷总氮全局变量.vi" "总氮校准信息"() -> (w380:T18)
              n211 = Index Array(array=w377, index=w378) -> (element=w375:T4)
              n212 = Bundle By Name(cluster=w384, "状态告警区"=w375, "平台试剂余量百分比"=w388, "关键参数"=w382, "关键参数改变"=w381, "校准信息"=w380, "校准信息改变"=w379) -> (w387:T11)
              n213 = Enqueue Element(queue=w386, element=w387) -> ()  [unwired: 2 in, 3 out]
            }
          }
        }
        frame 3 {
          (unwired) FALSE
          n214 = Get Queue Status(queue=w390) -> (queue out=w392:refnum<queue>, # elements in queue=w393:i32)  [unwired: 2 in, 6 out]
          n215 = Equal To 0?(x=w393) -> (x = 0?=w391:bool)
          n216 = case shown="真" w391 {
            tunnel: w392 -> [_ w405]
            tunnel: w389 -> [_ w404]
            frame False {
            }
            frame True {
              w395 = u16 3 items=["总磷"=1, "总氮"=2, "氨氮"=3, "磷酸盐"=4, "硝氮"=5, "亚硝氮"=6, "硅酸盐"=7, "硫化物"=8, "CODCr"=22]
              n217 = Unbundle By Name(w404) -> ("关键参数"=w403:T16)
              n218 = global read "VAR总磷总氮全局变量.vi" "氨氮关键参数"() -> (w401:T17)
              n219 = global read "VAR总磷总氮全局变量.vi" "状态告警区数组"() -> (w396:T7)
              n220 = global read "VAR总磷总氮全局变量.vi" "平台试剂余量百分比"() -> (w407:sgl)
              n221 = call "id参数转换.vi"("id"=w395) -> ("数组资源索引"=w397:i32)  [unwired: 9 in, 1 out]
              n222 = call "转换关键参数(子VI).vi"("参数"=w395, "总磷关键参数"=w401, "关键参数输入"=w403) -> ("关键参数输出"=w402:T16)  [unwired: 8 in]
              n223 = global read "VAR总磷总氮全局变量.vi" "氨氮关键参数改变"() -> (w400:bool)
              n224 = global read "VAR总磷总氮全局变量.vi" "氨氮校准信息改变"() -> (w398:bool)
              n225 = global read "VAR总磷总氮全局变量.vi" "氨氮校准信息"() -> (w399:T18)
              n226 = Index Array(array=w396, index=w397) -> (element=w394:T4)
              n227 = Bundle By Name(cluster=w404, "状态告警区"=w394, "平台试剂余量百分比"=w407, "关键参数"=w402, "关键参数改变"=w400, "校准信息"=w399, "校准信息改变"=w398) -> (w406:T12)
              n228 = Enqueue Element(queue=w405, element=w406) -> ()  [unwired: 2 in, 3 out]
            }
          }
        }
        frame 22 {
          n229 = Get Queue Status(queue=w409) -> (queue out=w411:refnum<queue>, # elements in queue=w412:i32)  [unwired: 2 in, 6 out]
          n230 = Equal To 0?(x=w412) -> (x = 0?=w410:bool)
          n231 = case shown="真" w410 {
            tunnel: w411 -> [_ w424]
            tunnel: w408 -> [_ w423]
            frame False {
            }
            frame True {
              w414 = u16 22 items=["总磷"=1, "总氮"=2, "氨氮"=3, "磷酸盐"=4, "硝氮"=5, "亚硝氮"=6, "硅酸盐"=7, "硫化物"=8, "CODCr"=22]
              n232 = Unbundle By Name(w423) -> ("关键参数"=w422:T16)
              n233 = global read "VAR总磷总氮全局变量.vi" "CODcr关键参数"() -> (w421:T17)
              n234 = global read "VAR总磷总氮全局变量.vi" "状态告警区数组"() -> (w415:T7)
              n235 = global read "VAR总磷总氮全局变量.vi" "CODCr关键参数改变"() -> (w419:bool)
              n236 = global read "VAR总磷总氮全局变量.vi" "CODCr校准信息改变"() -> (w417:bool)
              n237 = global read "VAR总磷总氮全局变量.vi" "平台试剂余量百分比"() -> (w426:sgl)
              n238 = call "id参数转换.vi"("id"=w414) -> ("数组资源索引"=w416:i32)  [unwired: 9 in, 1 out]
              n239 = call "转换关键参数(子VI).vi"("参数"=w414, "总磷关键参数"=w421, "关键参数输入"=w422) -> ("关键参数输出"=w420:T16)  [unwired: 8 in]
              n240 = global read "VAR总磷总氮全局变量.vi" "CODCr校准信息"() -> (w418:T18)
              n241 = Index Array(array=w415, index=w416) -> (element=w413:T4)
              n242 = Bundle By Name(cluster=w423, "状态告警区"=w413, "平台试剂余量百分比"=w426, "关键参数"=w420, "关键参数改变"=w419, "校准信息"=w418, "校准信息改变"=w417) -> (w425:T9)
              n243 = Enqueue Element(queue=w424, element=w425) -> ()  [unwired: 2 in, 3 out]
            }
          }
        }
        frame 21 {
          (unwired) FALSE
          n244 = Get Queue Status(queue=w428) -> (queue out=w430:refnum<queue>, # elements in queue=w431:i32)  [unwired: 2 in, 6 out]
          n245 = Equal To 0?(x=w431) -> (x = 0?=w429:bool)
          n246 = case shown="真" w429 {
            tunnel: w430 -> [_ w443]
            tunnel: w427 -> [_ w442]
            frame False {
            }
            frame True {
              w433 = u16 21 items=["总磷"=1, "总氮"=2, "氨氮"=3, "磷酸盐"=4, "硝氮"=5, "亚硝氮"=6, "硅酸盐"=7, "硫化物"=8, "CODMn"=21, "CODCr"=22, "氟化物"=50]
              n247 = Unbundle By Name(w442) -> ("关键参数"=w441:T16)
              n248 = global read "VAR总磷总氮全局变量.vi" "CODMn关键参数"() -> (w440:T17)
              n249 = global read "VAR总磷总氮全局变量.vi" "状态告警区数组"() -> (w434:T7)
              n250 = global read "VAR总磷总氮全局变量.vi" "CODmn关键参数改变"() -> (w438:bool)
              n251 = global read "VAR总磷总氮全局变量.vi" "CODMn校准信息改变"() -> (w436:bool)
              n252 = global read "VAR总磷总氮全局变量.vi" "平台试剂余量百分比"() -> (w445:sgl)
              n253 = call "id参数转换.vi"("id"=w433) -> ("数组资源索引"=w435:i32)  [unwired: 9 in, 1 out]
              n254 = call "转换关键参数(子VI).vi"("参数"=w433, "总磷关键参数"=w440, "关键参数输入"=w441) -> ("关键参数输出"=w439:T16)  [unwired: 8 in]
              n255 = global read "VAR总磷总氮全局变量.vi" "CODMn校准信息"() -> (w437:T18)
              n256 = Index Array(array=w434, index=w435) -> (element=w432:T4)
              n257 = Bundle By Name(cluster=w442, "状态告警区"=w432, "平台试剂余量百分比"=w445, "关键参数"=w439, "关键参数改变"=w438, "校准信息"=w437, "校准信息改变"=w436) -> (w444:T9)
              n258 = Enqueue Element(queue=w443, element=w444) -> ()  [unwired: 2 in, 3 out]
            }
          }
        }
        frame Default {
        }
      }
    }
  }
